vi "Main UI - Cylinder.vi"() -> ()   [LabVIEW 2015]
doc: "User interface for 64 pressure multiplexer system designed by Paul Nathan, 02/2016"
uses:
  Ctls/System status.ctl
  Ctls/Environmental state values.ctl
  Ctls/Inertial state values.ctl
  Ctls/AccelGyro constants.ctl
  Ctls/Pressure sensor constants.ctl
  Ctls/Cmd str.ctl
  Ctls/All state values (for datalog).ctl
  Ctls/Data values, Mode 0 (for datalog).ctl
  Ctls/Data values, Mode 1 (for datalog).ctl
panel:
  in  "Main tabs":T1(tab)
  out "ASCII done":bool caption="Done"
  in  "Write ASCII datalog":bool
  in  "Datalog name (without extension)":string="Log001"
  in  "Write interval (s)":u32=10
  in  "Save data":bool
  in  "Datalog directory":path=path "C:/Datalogs"
  out "ACK 8":bool caption="ACK"
  out "ACK 7":bool caption="ACK"
  out "ACK 6":bool caption="ACK"
  out "AccelGyro constants":T2={"gyrRange"=125.0, "accRange"=2.0, "gx offset"=0.0, "gy offset"=0.0, "gz offset"=0.0, "ax offset"=0.0, "ay offset"=0.0, "az offset"=0.0, "axyz scale"=1.0} {"axyz scale" format="%#_4f"; "az offset" format="%#_4f"; "ay offset" format="%#_4f"; "ax offset" format="%#_4f"; "gz offset" format="%#_4f"; "gy offset" format="%#_4f"; "gx offset" format="%#_4f"; "gyrRange" format="%#_4f"; "accRange" format="%#_4f"}
  out "Faulty sensors":i32[](array[numeric])
  out "ACK 5":bool caption="ACK"
  in  "Stop UI":bool
  out "Active sensors":i32[](array[numeric])
  in  "Refresh sys. status":bool
  out "ACK 4":bool caption="ACK"
  in  "Apply settings 3":bool caption="Apply settings"
  in  "Gyro. rate (Hz)":u8(ring) items=["6.25", "12.5", "25", "50", "100", "200", "400", "800", "1600", "3200"]
  in  "Gyro. range (dps)":u8(ring) items=["+/- 125", "+/- 250", "+/- 500", "+/- 1000", "+/- 2000"]
  in  "Accel. rate (Hz)":u8(ring)=1 items=["3.125", "6.25", "12.5", "25", "50", "100", "200", "400", "800", "1600"]
  in  "Accel. range (g)":u8(ring) items=["+/- 2", "+/- 4", "+/- 8", "+/- 16"]
  out "Inertial state values":T3 {"w_z (dps)" format="%#_4f"; "a_y (g)" format="%#_4f"; "a_z (g)" format="%#_4f"; "w_y (dps)" format="%#_4f"; "a_x (g)" format="%#_4f"; "Sensor temp. (degC)" format="%#.2f"; "w_x (dps)" format="%#_4f"}
  out "Environmental state values":T4 {"Dew point (degC)" format="%#.2f"; "Density (kg/m^3)" format="%#.3f"; "Pressure alt. (m)" format="%#.2f"; "Density alt. (m)" format="%#.2f"; "Rel. Humidity (%)" format="%#.2f"; "P_atmos (Pa)" format="%#_6f"; "Sensor temp. (degC)" format="%#.2f"; "Thermistor (degC)" format="%#.2f"}
  out "System status":T5
  out "ACK 3":bool caption="ACK"
  in  "Apply settings 2":bool caption="Apply setting"
  in  "Max. num. sensors (override)":u8=64 max=64
  out "ACK 1":bool caption="ACK"
  in  "Env. period (ms)":i32=1000 min=0
  in  "Data mode":u8(ring) items=["P", "P & T"]
  out "ACK 2":bool caption="ACK"
  in  "Apply settings 1":bool caption="Apply settings"
  in  "Data rate (Hz)":dbl=100.0
  in  "Reset":bool
  in  "Main Power":bool
  in  "Serial port":refnum<visa-resource-name>="COM1"
  out "Error":errorcluster
  out "L_data (bytes)":u16
  out "Serial no.":u16 format="%04x"
  out "Active pressure sensor constants":T6[](array[typedef])
  in  "d.p":i16=4
  in  "Wait for HW trigger":bool
  out "Clock drift":bool
  in  "Display rate (Hz)":dbl=100.0 min=0.0
  in  "N samples":u32=1000
  in  "Finite samples":bool
  out "Sensor temperatures time trace (Mode \"P & T\" only)":sgl[][](graph)
  out "Pressures time trace":sgl[][](graph)
  in  "Stop streaming":bool
  in  "Start streaming":bool
  out "Stale samples flag":u8[][](graph)
  out "Samples acquired":u32
  out "ok":bool
  out "Fx (N)":sgl format="%#_4g"
  out "Fy (N)":sgl format="%#_4g"
  in  "Filename (full path)":path=path "C:/Datalogs/Cp_snapshot_001.txt"
  in  "Snapshot":bool
  out "Cp distribution (time averaged)":cluster{"x/c flap (sorted)":sgl[], sgl[]}[](graph)
  out "Uref (m/s)":sgl format="%#_4g"
  # "[time averaged at display rate]"
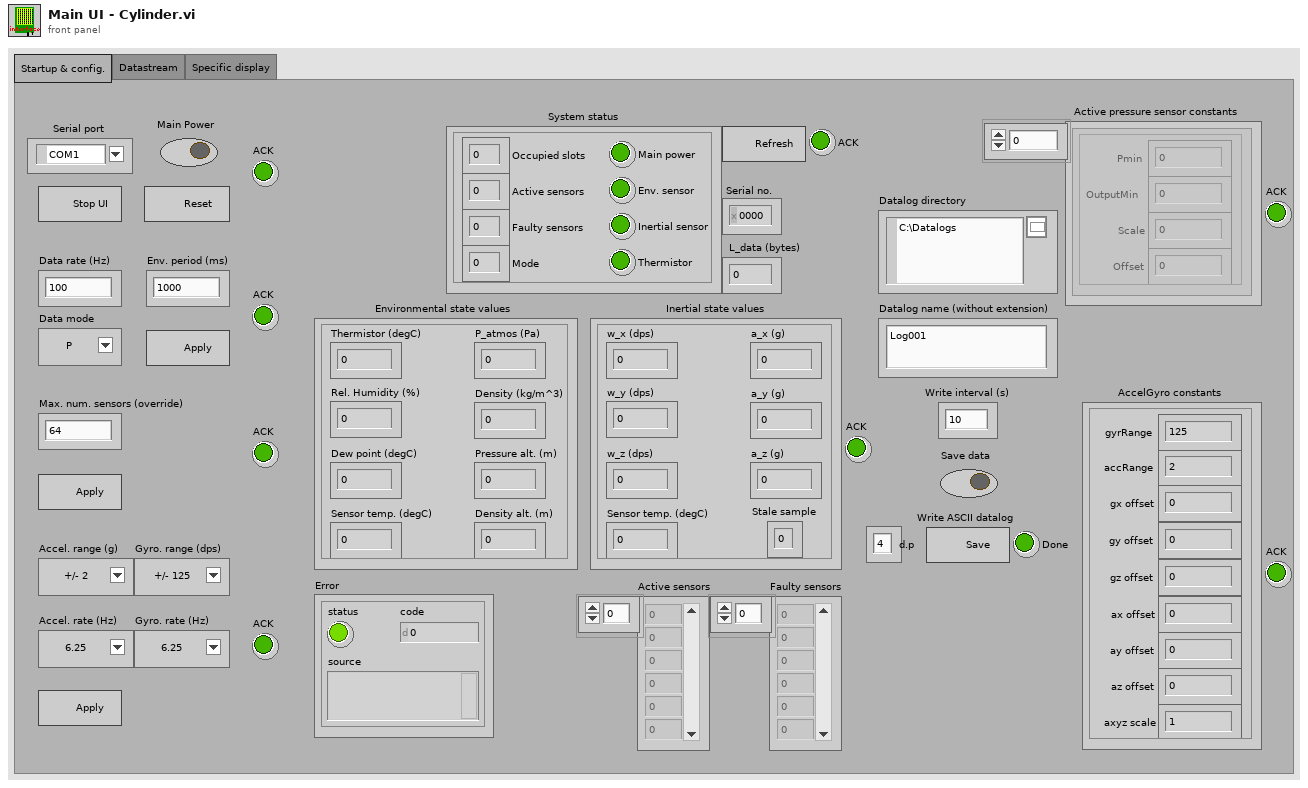
[diagram p1: front panel]
types:
  T1 = enum32{"Startup & config.", "Datastream", "Specific display"}
  T2 = typedef "AccelGyro constants.ctl" = cluster{"gyrRange":sgl, "accRange":sgl, "gx offset":sgl, "gy offset":sgl, "gz offset":sgl, "ax offset":sgl, "ay offset":sgl, "az offset":sgl, "axyz scale":sgl}
  T3 = typedef "Inertial state values.ctl" = cluster{"w_x (dps)":sgl, "w_y (dps)":sgl, "w_z (dps)":sgl, "a_x (g)":sgl, "a_y (g)":sgl, "a_z (g)":sgl, "Stale sample":u8, "Sensor temp. (degC)":sgl}
  T4 = typedef "Environmental state values.ctl" = cluster{"Thermistor (degC)":sgl, "Sensor temp. (degC)":sgl, "P_atmos (Pa)":sgl, "Rel. Humidity (%)":sgl, "Density (kg/m^3)":sgl, "Dew point (degC)":sgl, "Pressure alt. (m)":sgl, "Density alt. (m)":sgl}
  T5 = typedef "System status.ctl" = cluster{"Main power":bool, "Occupied slots":u8, "Active sensors":u8, "Faulty sensors":u8, "Env. sensor":bool, "Inertial sensor":bool, "Thermistor":bool, "Mode":u8}
  T6 = typedef "Pressure sensor constants.ctl" = cluster{"Pmin":sgl, "OutputMin":sgl, "Scale":sgl, "Offset":sgl}
  T7 = typedef "Cmd str.ctl" = string
  T8 = typedef "All state values (for datalog).ctl" = cluster{"Time Stamp":timestamp, "dt (ms)":i32, "Environmental state values":T4, "Inertial state values":T3}
  T9 = typedef "Data values, Mode 1 (for datalog).ctl" = cluster{"Time Stamp":timestamp, "dt (us)":sgl, "dt_warn":u8, "Pressures":sgl[], "Die temps.":sgl[], "Statuses":u8[]}
  T10 = typedef "Data values, Mode 0 (for datalog).ctl" = cluster{"Time Stamp":timestamp, "dt (us)":sgl, "dt_warn":u8, "Pressures":sgl[], "Statuses":u8[]}
  T11 = enum8{"Enabled", "Disabled", "Disabled and Grayed Out"}
  T12 = typedef "EEPROM page.ctl" = cluster{"Pmin (Pa)":sgl, "Pmax (Pa)":sgl, "maxCount":u16, "minCount":u16, "Poffset (Pa)":sgl}
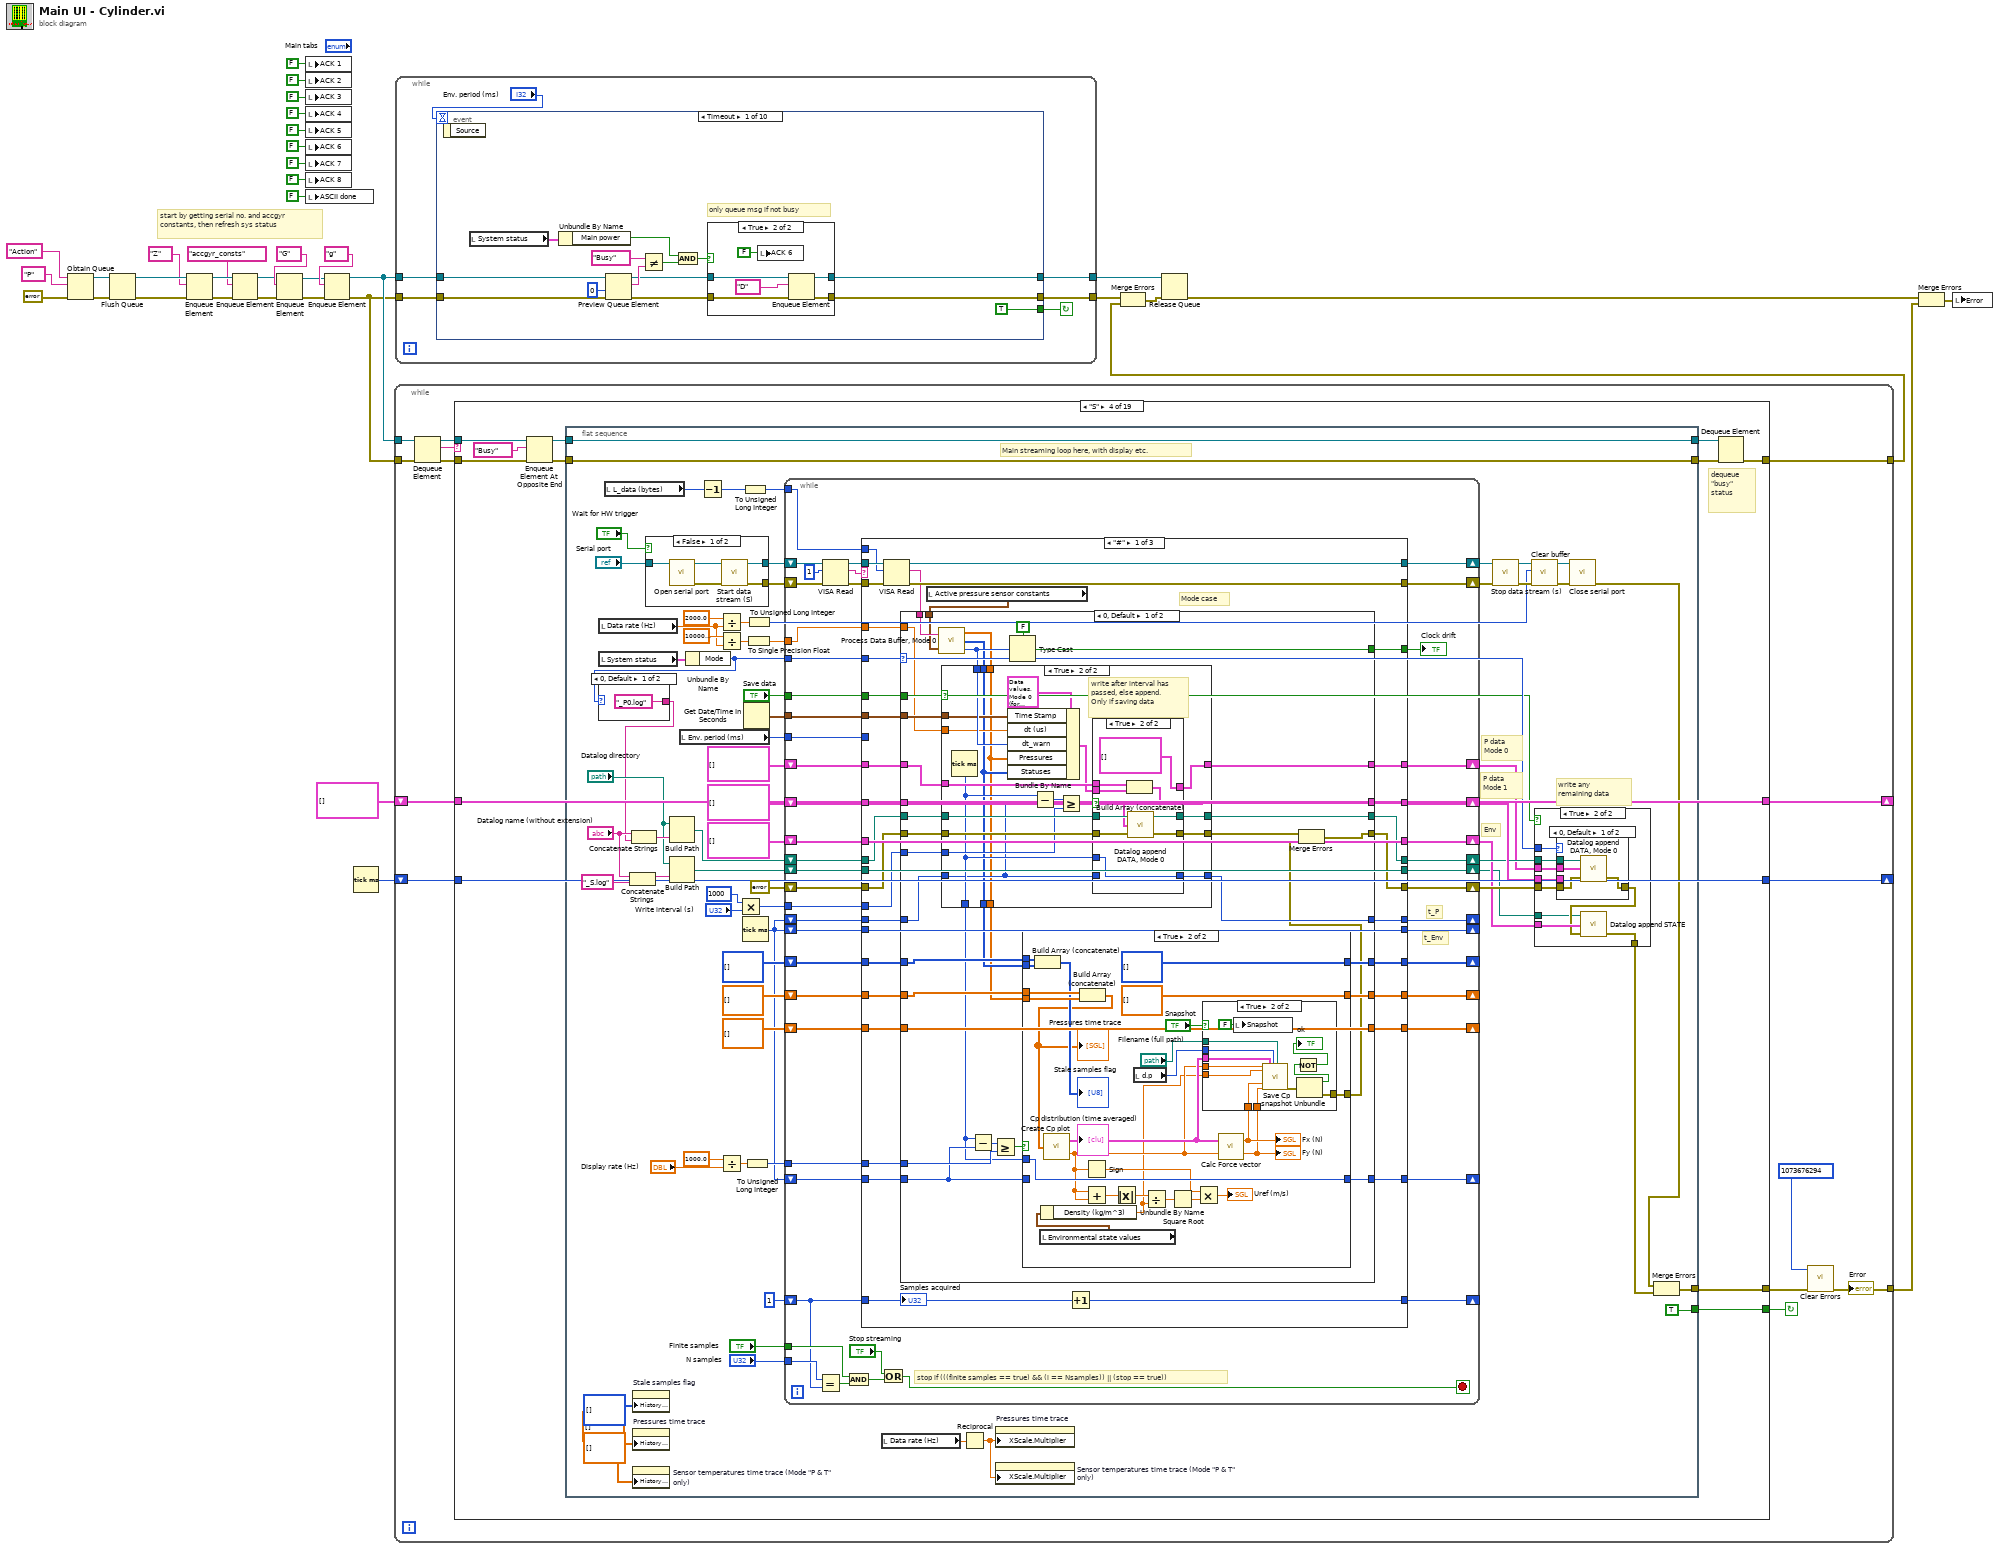
[diagram p0: block diagram]
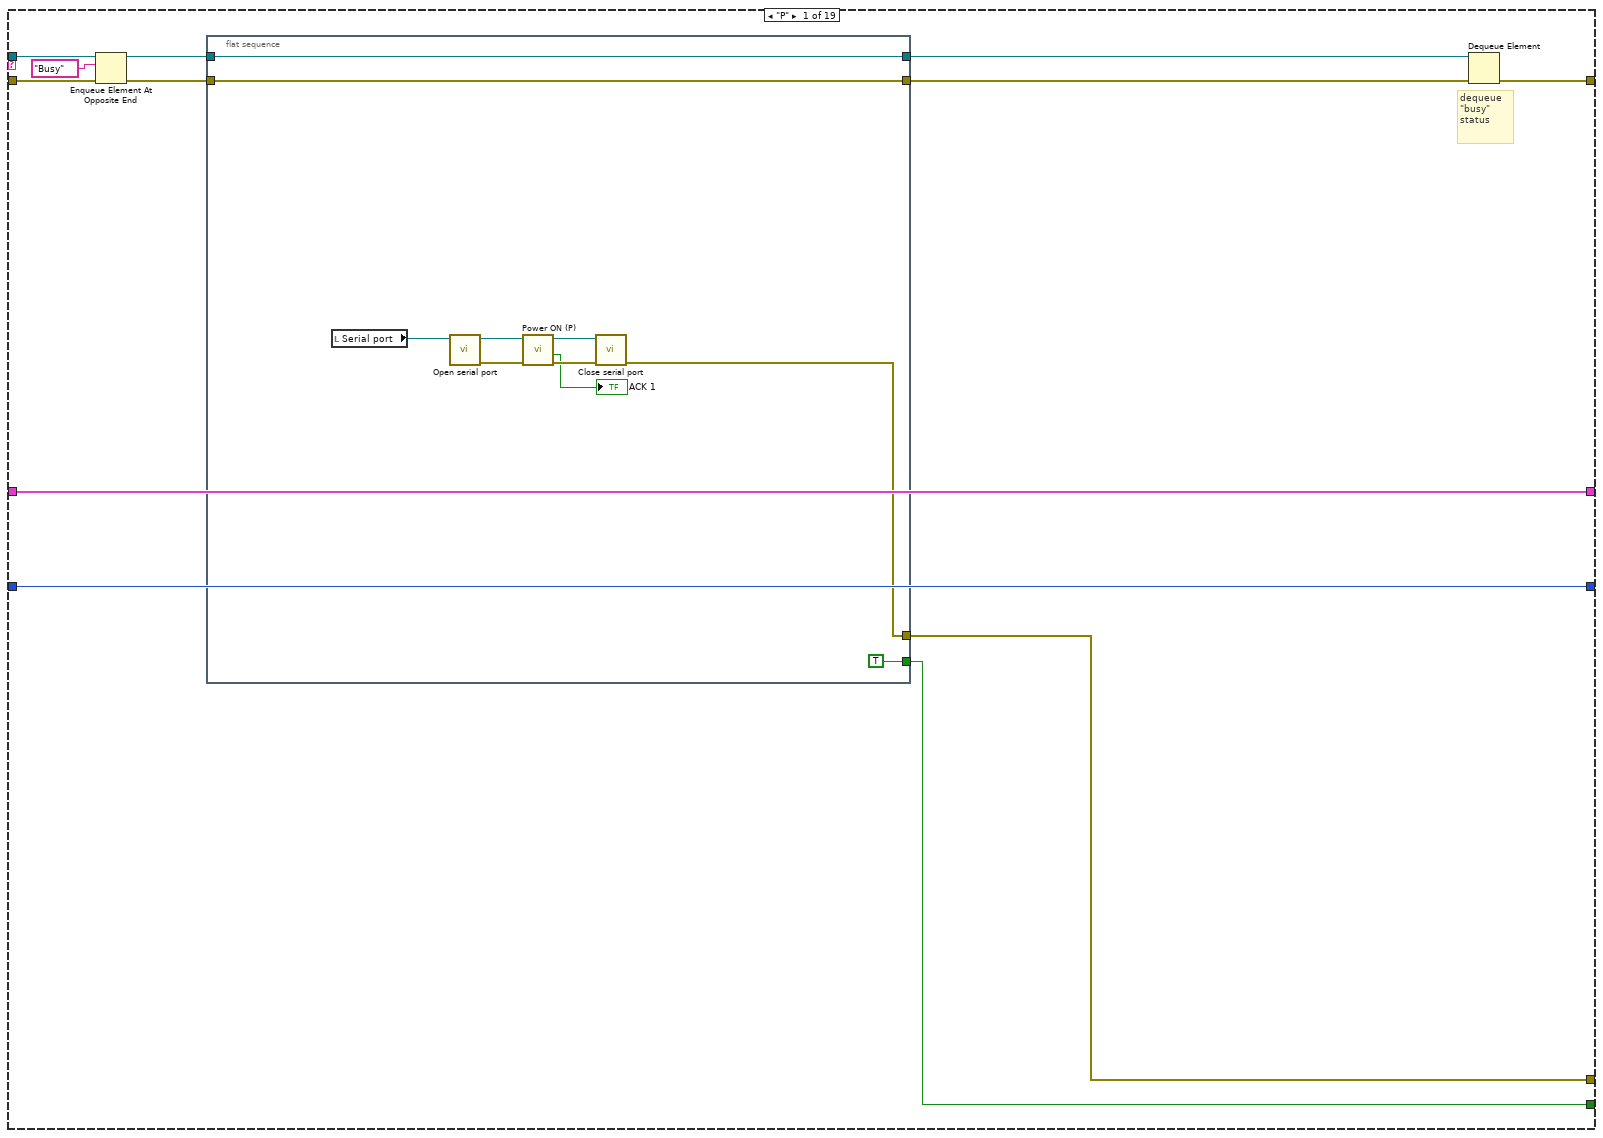
[diagram p2: hidden frame]
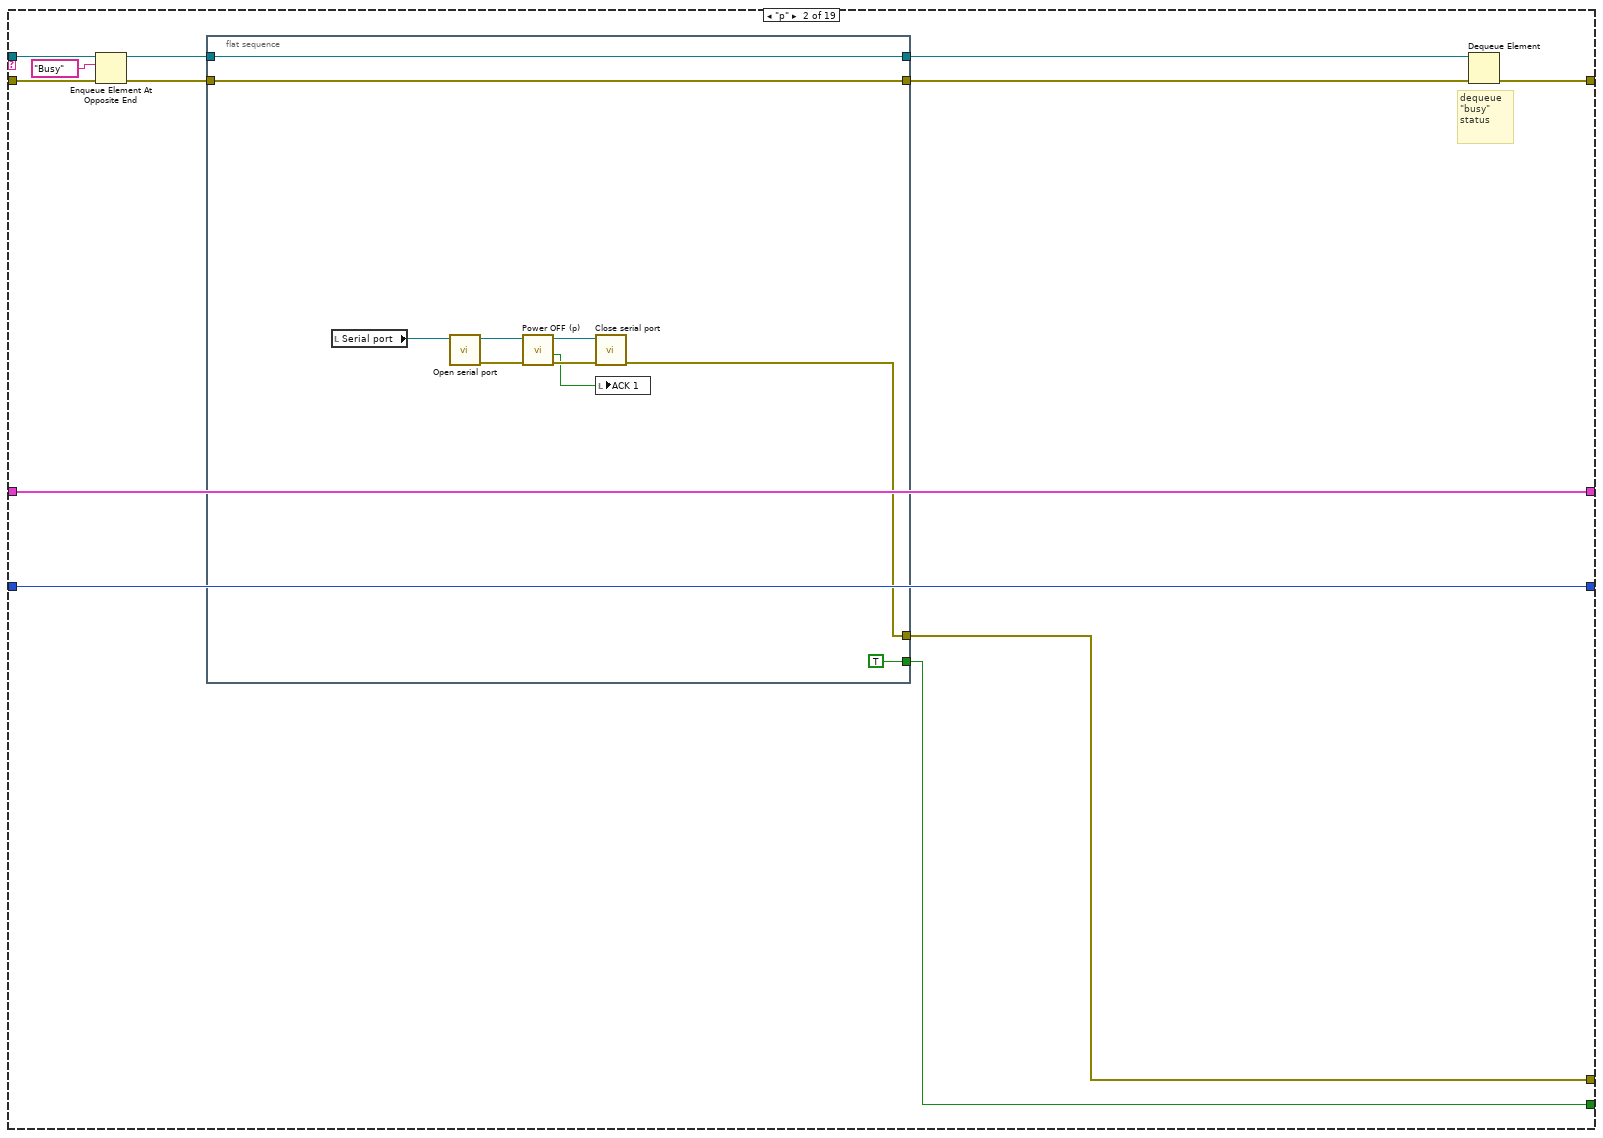
[diagram p3: hidden frame]
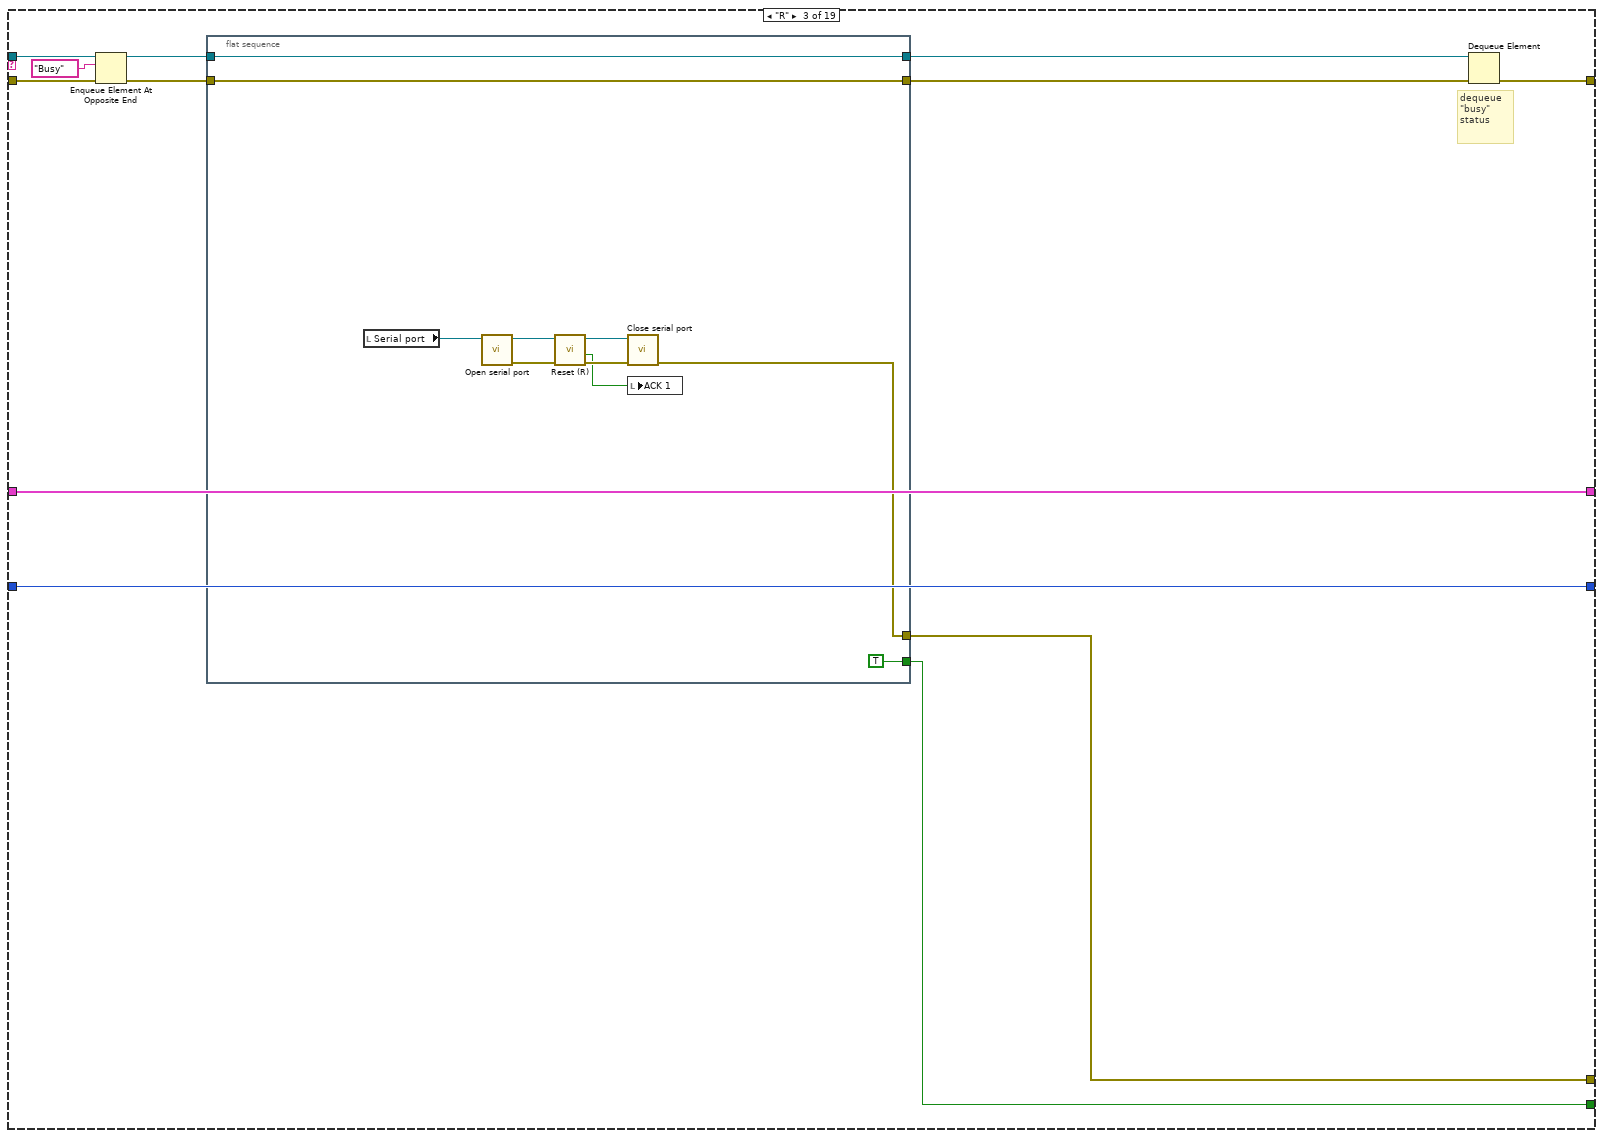
[diagram p4: hidden frame]
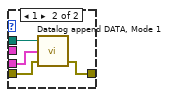
[diagram p6: hidden frame]
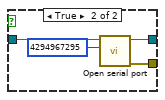
[diagram p7: hidden frame]
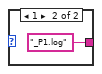
[diagram p8: hidden frame]
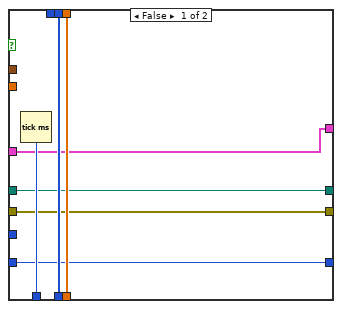
[diagram p9: hidden frame]
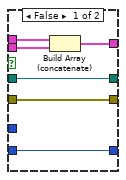
[diagram p10: hidden frame]
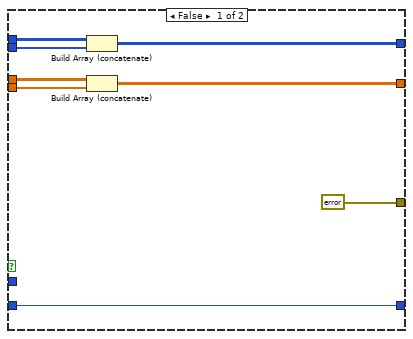
[diagram p11: hidden frame]
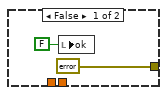
[diagram p12: hidden frame]
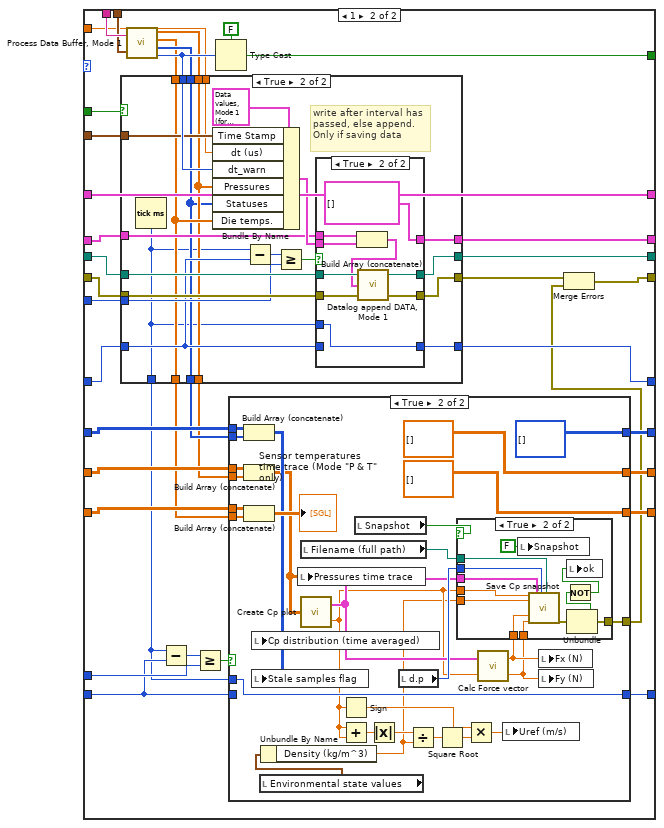
[diagram p13: hidden frame]
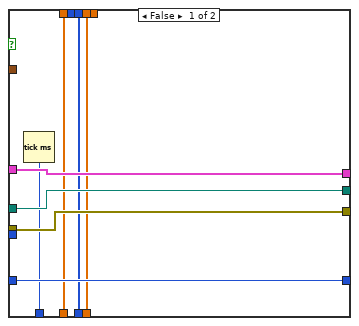
[diagram p14: hidden frame]
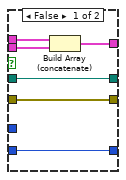
[diagram p15: hidden frame]
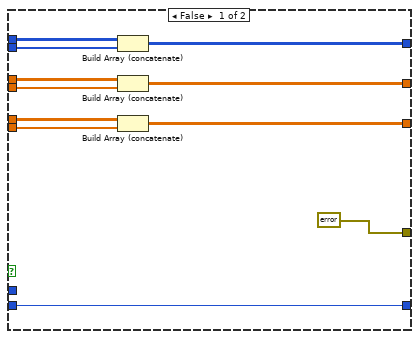
[diagram p16: hidden frame]
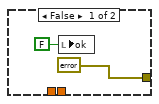
[diagram p17: hidden frame]
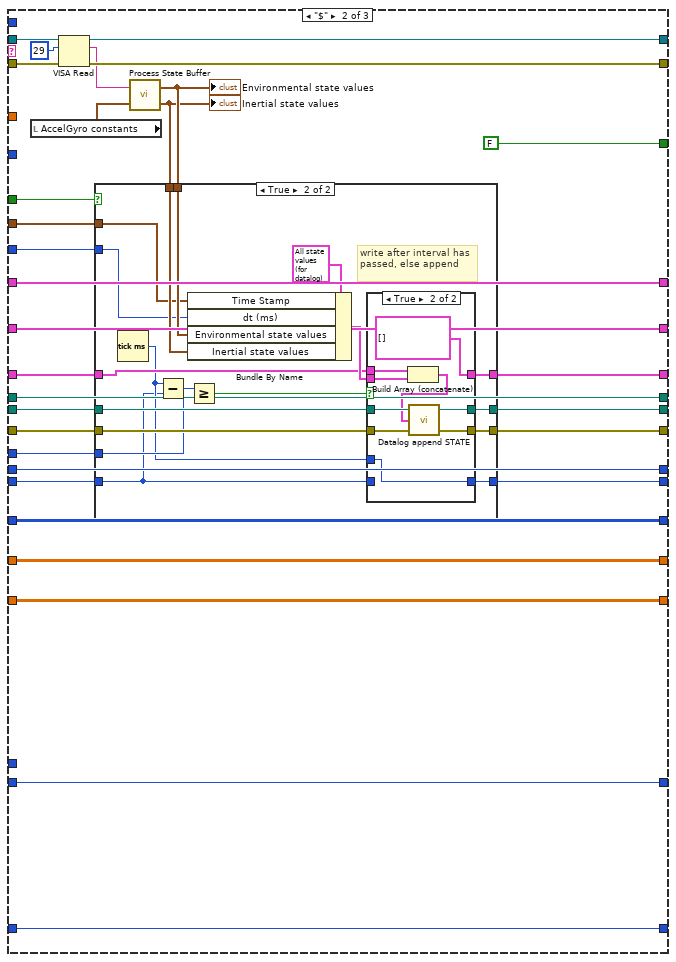
[diagram p18: hidden frame]
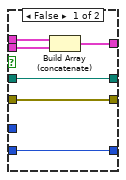
[diagram p20: hidden frame]
diagram:
  # "start by getting serial no. and accgyr constants, then refresh sys status"
  n1 = Obtain Queue(name (unnamed)="Action", element data type=T7 "P" ("Cmd"), error in (no error)=errorcluster {"status"=FALSE, "code"=0, "source"=""}) -> (queue out=w36:refnum<queue>, error out=w35:errorcluster)  [unwired: 2 in, 1 out]
  n2 = Flush Queue(queue=w36, error in (no error)=w35) -> (queue out=w28:refnum<queue>, error out=w27:errorcluster)  [unwired: 1 out]
  n3 = Enqueue Element(queue=w28, element=T7 "Z", error in (no error)=w27) -> (queue out=w25:refnum<queue>, error out=w24:errorcluster)  [unwired: 1 in, 1 out]
  n4 = Enqueue Element(queue=w25, element=T7 "accgyr_consts", error in (no error)=w24) -> (queue out=w12:refnum<queue>, error out=w11:errorcluster)  [unwired: 1 in, 1 out]
  n5 = Enqueue Element(queue=w12, element=T7 "G" ("Cmd"), error in (no error)=w11) -> (queue out=w14:refnum<queue>, error out=w15:errorcluster)  [unwired: 1 in, 1 out]
  n6 = local write "ACK 1"(FALSE ("ACK 8")) -> ()
  n7 = local write "ACK 2"(FALSE ("ACK 6")) -> ()
  n8 = local write "ACK 3"(FALSE ("ACK 8")) -> ()
  n9 = local write "ACK 4"(FALSE ("Done")) -> ()
  n10 = local write "ACK 5"(FALSE ("ACK 8")) -> ()
  n11 = local write "ACK 6"(FALSE ("ACK 6")) -> ()
  n12 = local write "ACK 7"(FALSE ("ACK 6")) -> ()
  n13 = local write "ACK 8"(FALSE ("ACK 8")) -> ()
  n14 = local write "ASCII done"(FALSE ("Done")) -> ()
  n15 = Enqueue Element(queue=w14, element=T7 "g" ("Cmd"), error in (no error)=w15) -> (queue out=w10:refnum<queue>, error out=w9:errorcluster)  [unwired: 1 in, 1 out]
  n16 = Tick Count (ms)() -> (millisecond timer value=w20:u32)
  n17 = while {
    tunnel: w9 -> [w50]
    tunnel: w10 -> [w51]
    tunnel: [w47] -> w30
    shift-right: [w44] -> _
    shift-left: T8[] [] -> [w43]
    tunnel: [w38] -> w18
    shift-right: [w41] -> _
    shift-left: w20 -> [w42]
    stop <- w46 continue-if-true
    n18 = Dequeue Element(queue=w51, error in (no error)=w50) -> (queue out=w49:refnum<queue>, element=w45:T7, error out=w48:errorcluster)  [unwired: 1 in, 1 out]
    n19 = case shown="\"S\"" w45 {
      tunnel: w49 -> [w63 w85 w107 w129 w664 w689 w713 w737 w761 w789 w826 w848 w870 w909 w933 w1006 w1038 w1066 _]
      tunnel: w48 -> [w62 w84 w106 w128 w663 w688 w712 w736 w760 w788 w825 w847 w869 w908 w932 w1005 w1037 w1065 w1135]
      tunnel: [w57 w79 w101 w123 w658 w683 w707 w731 w755 w783 w820 w842 w864 w903 w927 w1000 w1032 w1060 w1135] -> w47
      tunnel: [w56 w78 w100 w122 w657 w682 w706 w730 w754 w782 w819 w841 w863 w902 w926 w999 w1031 w1059 FALSE] -> w46
      tunnel: [w55 w77 w99 w121 w656 w681 w705 w729 w753 w781 w818 w840 w862 w901 w925 w998 w1030 w1058 errorcluster {"status"=FALSE, "code"=0, "source"=""} ("Error out")] -> w39
      tunnel: [w53 w75 w97 w118 w654 w679 w703 w727 w751 w779 w816 w838 w860 w899 w923 w995 w1028 w1056 w1132] -> w44
      tunnel: w43 -> [w53 w75 w97 w118 w654 w679 w703 w727 w751 w779 w816 w838 w860 w899 w922 w995 w1028 w1056 w1132]
      tunnel: w42 -> [w52 w74 w96 w119 w653 w678 w702 w726 w750 w778 w815 w837 w859 w898 w921 w996 w1027 w1055 w1131]
      tunnel: [w52 w74 w96 w119 w653 w678 w702 w726 w750 w778 w815 w837 w859 w898 w920 w996 w1027 w1055 w1131] -> w41
      frame "P" {
        # "dequeue \"busy\" status"
        n20 = Enqueue Element At Opposite End(queue=w63, element=T7 "Busy" ("Cmd"), error in (no error)=w62) -> (queue out=w61:refnum<queue>, error out=w60:errorcluster)  [unwired: 1 in, 1 out]
        n21 = flat-sequence {
          tunnel: w61 -> [w73]
          tunnel: w60 -> [w72]
          tunnel: [w73] -> w59
          tunnel: [w72] -> w58
          tunnel: [TRUE] -> w56
          tunnel: [w66] -> w55
          frame #0 {
            n22 = local read "Serial port"() -> (w65:refnum<visa-resource-name>)
            n23 = call "Open serial port.vi"("VISA resource name"=w65) -> ("Error out"=w69:errorcluster, "VISA resource name out"=w70:refnum<visa-resource-name>)  [unwired: 9 in]
            n24 = call "Power ON (P).vi"("Error In"=w69, "VISA resource name in"=w70) -> ("Error out"=w68:errorcluster, "ACK"=→"ACK 1":bool, "VISA resource name out"=w67:refnum<visa-resource-name>)  [unwired: 7 in]
            n25 = call "Close serial port.vi"("Error in"=w68, "VISA resource name"=w67) -> ("Error out"=w66:errorcluster)  [unwired: 9 in]
          }
        }
        n26 = Dequeue Element(queue=w59, error in (no error)=w58) -> (error out=w57:errorcluster)  [unwired: 1 in, 3 out]
      }
      frame "p" {
        # "dequeue \"busy\" status"
        n27 = Enqueue Element At Opposite End(queue=w85, element=T7 "Busy" ("Cmd"), error in (no error)=w84) -> (queue out=w83:refnum<queue>, error out=w82:errorcluster)  [unwired: 1 in, 1 out]
        n28 = flat-sequence {
          tunnel: w83 -> [w95]
          tunnel: w82 -> [w94]
          tunnel: [w95] -> w81
          tunnel: [w94] -> w80
          tunnel: [TRUE] -> w78
          tunnel: [w88] -> w77
          frame #0 {
            n29 = local read "Serial port"() -> (w86:refnum<visa-resource-name>)
            n30 = call "Open serial port.vi"("VISA resource name"=w86) -> ("Error out"=w91:errorcluster, "VISA resource name out"=w92:refnum<visa-resource-name>)  [unwired: 9 in]
            n31 = call "Power OFF (p).vi"("Error In"=w91, "VISA resource name in"=w92) -> ("Error out"=w90:errorcluster, "ACK"=w87:bool, "VISA resource name out"=w89:refnum<visa-resource-name>)  [unwired: 7 in]
            n32 = call "Close serial port.vi"("Error in"=w90, "VISA resource name"=w89) -> ("Error out"=w88:errorcluster)  [unwired: 9 in]
            n33 = local write "ACK 1"(w87) -> ()
          }
        }
        n34 = Dequeue Element(queue=w81, error in (no error)=w80) -> (error out=w79:errorcluster)  [unwired: 1 in, 3 out]
      }
      frame "R" {
        # "dequeue \"busy\" status"
        n35 = Enqueue Element At Opposite End(queue=w107, element=T7 "Busy" ("Cmd"), error in (no error)=w106) -> (queue out=w105:refnum<queue>, error out=w104:errorcluster)  [unwired: 1 in, 1 out]
        n36 = flat-sequence {
          tunnel: w105 -> [w117]
          tunnel: w104 -> [w116]
          tunnel: [w117] -> w103
          tunnel: [w116] -> w102
          tunnel: [TRUE] -> w100
          tunnel: [w112] -> w99
          frame #0 {
            n37 = local read "Serial port"() -> (w110:refnum<visa-resource-name>)
            n38 = call "Open serial port.vi"("VISA resource name"=w110) -> ("Error out"=w108:errorcluster, "VISA resource name out"=w109:refnum<visa-resource-name>)  [unwired: 9 in]
            n39 = call "Reset (R).vi"("Error In"=w108, "VISA resource name in"=w109) -> ("Error out"=w114:errorcluster, "ACK"=w111:bool, "VISA resource name out"=w113:refnum<visa-resource-name>)  [unwired: 7 in]
            n40 = call "Close serial port.vi"("Error in"=w114, "VISA resource name"=w113) -> ("Error out"=w112:errorcluster)  [unwired: 9 in]
            n41 = local write "ACK 1"(w111) -> ()
          }
        }
        n42 = Dequeue Element(queue=w103, error in (no error)=w102) -> (error out=w101:errorcluster)  [unwired: 1 in, 3 out]
      }
      frame "S" {
        # "dequeue \"busy\" status"
        n43 = Enqueue Element At Opposite End(queue=w129, element=T7 "Busy" ("Cmd"), error in (no error)=w128) -> (queue out=w127:refnum<queue>, error out=w126:errorcluster)  [unwired: 1 in, 1 out]
        n44 = flat-sequence {
          tunnel: w127 -> [w197]
          tunnel: w126 -> [w196]
          tunnel: [w197] -> w125
          tunnel: [w196] -> w124
          tunnel: [TRUE] -> w122
          tunnel: [w183] -> w121
          frame #0 {
            # "Env"
            # "P data Mode 1"
            # "P data Mode 0"
            # "write any remaining data"
            # "Main streaming loop here, with display etc."
            n45 = local read "Data rate (Hz)"() -> (w158:dbl)
            n46 = local read "System status"() -> (w155:T5)
            n47 = local read "L_data (bytes)"() -> (w162:u16)
            n48 = Concatenate Strings("Datalog name (without extension)", "_S.log" ("string")) -> (w169:string)
            n49 = property on="Stale samples flag" class="WFChart (strict)"("History Data"=u8[][] []) -> ()  [unwired: 2 in, 2 out]
            n50 = property on="Pressures time trace" class="WFChart (strict)"("History Data"=sgl[][] []) -> ()  [unwired: 2 in, 2 out]
            n51 = property on="Sensor temperatures time trace (Mode \"P & T\" only)" class="WFChart (strict)"("History Data"=sgl[][] []) -> ()  [unwired: 2 in, 2 out]
            n52 = case shown="False" "Wait for HW trigger" {
              tunnel: [w218 w222] -> w194
              tunnel: [w217 w223] -> w193
              tunnel: "Serial port" -> [w216 w224]
              frame False {
                n53 = call "Open serial port.vi"("VISA resource name"=w216) -> ("Error out"=w219:errorcluster, "VISA resource name out"=w220:refnum<visa-resource-name>)  [unwired: 9 in]
                n54 = call "Start data stream (S).vi"("VISA resource name in"=w220, "Error In"=w219) -> ("VISA resource name out"=w217:refnum<visa-resource-name>, "Error out"=w218:errorcluster)  [unwired: 7 in]
              }
              frame True {
                n55 = call "Open serial port.vi"("timeout (ms)"=u32 4294967295, "VISA resource name"=w224) -> ("Error out"=w222:errorcluster, "VISA resource name out"=w223:refnum<visa-resource-name>)  [unwired: 8 in]
              }
            }
            n56 = Build Path(base path="Datalog directory", name or relative path=w169) -> (appended path=w165:path)
            n57 = local read "Env. period (ms)"() -> (w160:i32)
            n58 = Unbundle By Name(w155) -> ("Mode"=w140:u8)
            n59 = case shown="0, Default" w140 {
              tunnel: ["_P0.log" ("string") "_P1.log" ("string")] -> w154
              frame 0, Default {
              }
              frame 1 {
              }
            }
            n60 = Concatenate Strings("Datalog name (without extension)", w154) -> (w177:string)
            n61 = Build Path(base path="Datalog directory", name or relative path=w177) -> (appended path=w166:path)
            n62 = Decrement(x=w162) -> (x-1=w144:u16)
            n63 = Divide(x=2000.0 ("y"), y=w158) -> (x/y=w186:dbl)
            n64 = Divide(x=1000000.0 ("y"), y=w158) -> (x/y=w157:dbl)
            n65 = Divide(x=1000.0, y="Display rate (Hz)") -> (x/y=w175:dbl)
            n66 = Multiply(x=u32 1000, y="Write interval (s)") -> (x*y=w179:u32)
            n67 = To Unsigned Long Integer(number=w144) -> (unsigned 32bit integer=w161:u32)
            n68 = Tick Count (ms)() -> (millisecond timer value=w145:u32)
            n69 = Get Date/Time In Seconds() -> (seconds since 1Jan1904=w192:timestamp)
            n70 = To Unsigned Long Integer(number=w175) -> (unsigned 32bit integer=w172:u32)
            n71 = To Unsigned Long Integer(number=w186) -> (unsigned 32bit integer=w185:u32)
            n72 = To Single Precision Float(number=w157) -> (single precision float=w156:sgl)
            n73 = while {
              shift-right: [w269] -> w189
              shift-left: w193 -> [w274]
              shift-right: [w268] -> w190
              shift-left: w194 -> [w275]
              tunnel: w192 -> [w267]
              shift-right: [w266] -> w142
              shift-left: errorcluster {"status"=FALSE, "code"=0, "source"=""} ("Error out") -> [w265]
              tunnel: "Finite samples" -> [w262]
              tunnel: "N samples" -> [w264]
              tunnel: "Save data" -> [w258]
              shift-right: [w256] -> w136
              shift-left: w165 -> [w257]
              shift-right: [w255] -> w138
              shift-left: T8[] [] -> [w254]
              tunnel: w179 -> [w252]
              shift-right: [w247] -> _
              shift-left: w145 -> [w253]
              tunnel: w172 -> [w236]
              shift-right: [w250] -> w141
              shift-left: w166 -> [w251]
              shift-right: [w248] -> _
              shift-left: w145 -> [w249]
              shift-right: [w243] -> w143
              shift-left: T9[] [] -> [w245]
              shift-right: [w244] -> w139
              shift-left: T10[] [] -> [w246]
              tunnel: w161 -> [w242]
              tunnel: w160 -> [w241]
              tunnel: w156 -> [w240]
              tunnel: w140 -> [w229]
              shift-right: [w238] -> _
              shift-left: w145 -> [w237]
              shift-right: [w235] -> _
              shift-left: sgl[][] [] -> [w232]
              shift-right: [w234] -> _
              shift-left: u8[][] [] -> [w233]
              shift-right: [w231] -> _
              shift-left: sgl[][] [] -> [w230]
              shift-right: [w228] -> _
              shift-left: u32 1 ("x") -> [w227]
              stop <- w259 stop-if-true
              # "t_Env"
              # "t_P"
              # "stop if (((finite samples == true) && (i == Nsamples)) || (stop == true))"
              n74 = Equal?(x=w264, y=w227) -> (x = y?=w263:bool)
              n75 = VISA Read(VISA resource name=w274, byte count=u32 1, error in (no error)=w275) -> (VISA resource name out=w271:refnum<visa-resource-name>, read buffer=w272:string, error out=w270:errorcluster)  [unwired: 1 out]
              n76 = And(x=w262, y=w263) -> (x .and. y?=w260:bool)
              n77 = case shown="\"#\"" w272 {
                tunnel: w271 -> [w310 w598 w652]
                tunnel: w270 -> [w309 w597 w651]
                tunnel: [w307 w595 w652] -> w269
                tunnel: [w306 w596 w651] -> w268
                tunnel: w267 -> [w303 w592 _]
                tunnel: [w289 w591 w650] -> w266
                tunnel: w265 -> [w299 w590 w650]
                tunnel: w258 -> [w278 w589 _]
                tunnel: w257 -> [w312 w588 w649]
                tunnel: [w312 w587 w649] -> w256
                tunnel: [w311 w586 w648] -> w255
                tunnel: w254 -> [w311 w585 w648]
                tunnel: w253 -> [w294 w578 w645]
                tunnel: w252 -> [w296 w584 _]
                tunnel: [w295 w583 w646] -> w248
                tunnel: w251 -> [w300 w580 w647]
                tunnel: [w288 w580 w647] -> w250
                tunnel: w249 -> [w295 w579 w646]
                tunnel: [w298 w578 w645] -> w247
                tunnel: w246 -> [w302 w577 w643]
                tunnel: w245 -> [w291 w576 w644]
                tunnel: [w301 w577 w643] -> w244
                tunnel: [w290 w576 w644] -> w243
                tunnel: w242 -> [w308 _ _]
                tunnel: w241 -> [_ w575 _]
                tunnel: w240 -> [w297 _ _]
                tunnel: [w293 FALSE ("Clock drift") FALSE ("Clock drift")] -> w239
                tunnel: w229 -> [w292 _ _]
                tunnel: [w287 w573 w641] -> w238
                tunnel: w237 -> [w286 w573 w641]
                tunnel: w236 -> [w285 _ _]
                tunnel: [w284 w571 w639] -> w235
                tunnel: w232 -> [w283 w571 w639]
                tunnel: [w282 w572 w640] -> w234
                tunnel: w233 -> [w281 w572 w640]
                tunnel: [w280 w570 w638] -> w231
                tunnel: w230 -> [w279 w570 w638]
                tunnel: [w277 w569 w637] -> w228
                tunnel: w227 -> [w276 w569 w637]
                frame "#" {
                  # "Mode case"
                  n78 = VISA Read(VISA resource name=w310, byte count=w308, error in (no error)=w309) -> (VISA resource name out=w307:refnum<visa-resource-name>, read buffer=w305:string, error out=w306:errorcluster)  [unwired: 1 out]
                  n79 = local read "Active pressure sensor constants"() -> (w304:T6[])
                  n80 = case shown="0, Default" w292 {
                    tunnel: w305 -> [w346 w471]
                    tunnel: w304 -> [w345 w470]
                    tunnel: w303 -> [w342 w467]
                    tunnel: w302 -> [w341 w472]
                    tunnel: [w340 w472] -> w301
                    tunnel: w300 -> [w339 w466]
                    tunnel: w299 -> [w338 w465]
                    tunnel: [w337 w464] -> w298
                    tunnel: w297 -> [w336 w463]
                    tunnel: w296 -> [w335 w462]
                    tunnel: w294 -> [w320 w461]
                    tunnel: [w334 w460] -> w293
                    tunnel: w291 -> [w347 w459]
                    tunnel: [w347 w458] -> w290
                    tunnel: [w313 w437] -> w289
                    tunnel: [w333 w457] -> w288
                    tunnel: [w332 w451] -> w287
                    tunnel: w286 -> [w329 w447]
                    tunnel: w285 -> [w331 w448]
                    tunnel: [w326 w455] -> w284
                    tunnel: w283 -> [w325 w453]
                    tunnel: [w323 w456] -> w282
                    tunnel: w281 -> [w322 w454]
                    tunnel: [w321 w445] -> w280
                    tunnel: w279 -> [w321 w443]
                    tunnel: w278 -> [w317 w442]
                    frame 0, Default {
                      n81 = call "Process Data Buffer, Mode 0.vi"("DATA_Buffer excluding '#' [1...N]"=w346, "P constants"=w345) -> ("Pressures"=w327:sgl[], "Statuses"=w324:u8[], "dt_warn"=w343:u8)
                      n82 = case shown="True" w317 {
                        tunnel: w343 -> [_ w372]
                        tunnel: w342 -> [_ w371]
                        tunnel: w341 -> [w349 w370]
                        tunnel: [w349 w368] -> w340
                        tunnel: w339 -> [w350 w367]
                        tunnel: w338 -> [w351 w366]
                        tunnel: [w348 w365] -> w337
                        tunnel: w336 -> [_ w364]
                        tunnel: w335 -> [_ w361]
                        tunnel: [w351 w360] -> w315
                        tunnel: [w350 w359] -> w333
                        tunnel: [w354 w358] -> w316
                        tunnel: w327 -> [w352 w355]
                        tunnel: w324 -> [w353 w356]
                        tunnel: w320 -> [w348 w357]
                        tunnel: [w353 w356] -> w319
                        tunnel: [w352 w355] -> w318
                        frame False {
                          n83 = Tick Count (ms)() -> (millisecond timer value=w354:u32)
                        }
                        frame True {
                          # "write after interval has passed, else append. Only if saving data"
                          n84 = Tick Count (ms)() -> (millisecond timer value=w358:u32)
                          n85 = Bundle By Name(cluster=T10 {"Time Stamp"=timestamp(3537581686.1176577 s since 1904-01-01), "dt (us)"=0.0, "dt_warn"=0, "Pressures"=[], "Statuses"=[]} ("P data (Mode 0)"), "Time Stamp"=w371, "dt (us)"=w364, "dt_warn"=w372, "Pressures"=w355, "Statuses"=w356) -> (w369:T10)
                          n86 = Subtract(x=w358, y=w357) -> (x-y=w363:u32)
                          n87 = Greater Or Equal?(x=w363, y=w361) -> (x >= y?=w362:bool)
                          n88 = case shown="True" w362 {
                            tunnel: [w375 w388] -> w360
                            tunnel: w366 -> [w375 w387]
                            tunnel: w367 -> [w376 w386]
                            tunnel: [w376 w385] -> w359
                            tunnel: w369 -> [w378 w384]
                            tunnel: w370 -> [w379 w383]
                            tunnel: [w377 T10[] []] -> w368
                            tunnel: w358 -> [_ w382]
                            tunnel: [w374 w382] -> w365
                            tunnel: w357 -> [w374 _]
                            frame False {
                              n89 = Build Array (concatenate)(w379, w378) -> (w377:T10[])
                            }
                            frame True {
                              n90 = Build Array (concatenate)(w383, w384) -> (w380:T10[])
                              n91 = call "Datalog append DATA, Mode 0.vi"("Datalog (Data) path"=w386, "Data (Mode 0)"=w380, "Error in"=w387) -> ("Path out"=w385:path, "Error out"=w388:errorcluster)  [unwired: 5 in]
                            }
                          }
                        }
                      }
                      n92 = Subtract(x=w316, y=w329) -> (x-y=w330:u32)
                      n93 = Greater Or Equal?(x=w330, y=w331) -> (x >= y?=w328:bool)
                      n94 = Type Cast(type=FALSE ("Clock drift"), x=w343) -> (*(type *) &x=w334:bool)
                      n95 = case shown="True" w328 {
                        tunnel: [w396 w421] -> w332
                        tunnel: w329 -> [w396 _]
                        tunnel: w316 -> [_ w421]
                        tunnel: w318 -> [w395 w419]
                        tunnel: [w394 sgl[][] []] -> w326
                        tunnel: w325 -> [w393 w420]
                        tunnel: w319 -> [w392 w416]
                        tunnel: [w391 u8[][] []] -> w323
                        tunnel: w322 -> [w390 w417]
                        tunnel: [errorcluster {"status"=FALSE, "code"=0, "source"=""} ("error out") w410] -> w314
                        frame False {
                          n96 = Build Array (concatenate)(w390, w392) -> (w391:u8[][])
                          n97 = Build Array (concatenate)(w393, w395) -> (w394:sgl[][])
                        }
                        frame True {
                          n98 = Build Array (concatenate)(w417, w416) -> (→"Stale samples flag":u8[][])
                          n99 = local read "Environmental state values"() -> (w408:T4)
                          n100 = Unbundle By Name(w408) -> ("Density (kg/m^3)"=w399:sgl)
                          n101 = Build Array (concatenate)(w420, w419) -> (w413:sgl[][])
                          "Pressures time trace" <- w413
                          n102 = call "Create Cp plot.vi"("Pressures in (cols = sensor, rows = time)"=w413) -> ("Cp against x/c"=w401:cluster{"x/c flap (sorted)":sgl[], sgl[]}[], "Pdyn ref (Pa)"=w400:sgl)
                          "Cp distribution (time averaged)" <- w401
                          n103 = Sign(1:w400) -> (0:w402:sgl)
                          n104 = Add(x=w400, y=w400) -> (x+y=w407:sgl)
                          n105 = Absolute Value(x=w407) -> (abs(x)=w405:sgl)
                          n106 = local read "d.p"() -> (w411:i16)
                          n107 = Divide(x=w405, y=w399) -> (x/y=w406:sgl)
                          n108 = Square Root(x=w406) -> (sqrt(x)=w403:sgl)
                          n109 = Multiply(x=w402, y=w403) -> (x*y=→"Uref (m/s)":sgl)
                          n110 = call "Calc Force vector.vi"("Pdyn ref (Pa)"=w400, "Cp distribution (time averaged)"=w401) -> ("Fy (N)"=w397:sgl, "Fx (N)"=w398:sgl)
                          "Fx (N)" <- w398
                          "Fy (N)" <- w397
                          n111 = case shown="True" "Snapshot" {
                            tunnel: "Filename (full path)" -> [_ w434]
                            tunnel: w401 -> [_ w433]
                            tunnel: w411 -> [_ w432]
                            tunnel: [errorcluster {"status"=FALSE, "code"=0, "source"=""} ("error out") w429] -> w410
                            tunnel: w400 -> [_ w430]
                            tunnel: w399 -> [_ w428]
                            tunnel: w398 -> [_ w427]
                            tunnel: w397 -> [_ w426]
                            frame False {
                              n112 = local write "ok"(FALSE ("ok")) -> ()
                            }
                            frame True {
                              n113 = local write "Snapshot"(FALSE ("Snapshot")) -> ()
                              n114 = call "Save Cp snapshot.vi"("Pdyn ref (Pa)"=w430, "rho ref (kg/m^3)"=w428, "Fx (N)"=w427, "Fy (N)"=w426, "Cp distribution (time averaged)"=w433, "d.p"=w432, "File Path"=w434) -> ("error out"=w429:errorcluster)  [unwired: 12 in]
                              n115 = Unbundle(w429) -> ("status"=w425:bool)  [unwired: 2 out]
                              n116 = Not(x=w425) -> (.not. x?=→"ok":bool)
                            }
                          }
                        }
                      }
                      n117 = Merge Errors(w315, w314) -> (w313:errorcluster)
                    }
                    frame 1 {
                      n118 = call "Process Data Buffer, Mode 1.vi"("DATA_Buffer excluding '#' [1...N]"=w471, "P constants"=w470) -> ("Pressures (Pa)"=w452:sgl[], "Sensor temps (degC)"=w444:sgl[], "Statuses"=w446:u8[], "dt_warn"=w468:u8)
                      n119 = case shown="True" w442 {
                        tunnel: w468 -> [_ w499]
                        tunnel: w467 -> [_ w498]
                        tunnel: w466 -> [w478 w496]
                        tunnel: w465 -> [w479 w495]
                        tunnel: [w480 w494] -> w464
                        tunnel: w463 -> [_ w493]
                        tunnel: w462 -> [_ w490]
                        tunnel: w461 -> [w480 w489]
                        tunnel: w459 -> [w477 w488]
                        tunnel: [w477 w487] -> w458
                        tunnel: [w479 w486] -> w436
                        tunnel: [w478 w485] -> w457
                        tunnel: w452 -> [w475 w483]
                        tunnel: w446 -> [w474 w482]
                        tunnel: w444 -> [w476 w484]
                        tunnel: [w476 w484] -> w441
                        tunnel: [w475 w483] -> w439
                        tunnel: [w474 w482] -> w440
                        tunnel: [w473 w481] -> w438
                        frame False {
                          n120 = Tick Count (ms)() -> (millisecond timer value=w473:u32)
                        }
                        frame True {
                          # "write after interval has passed, else append. Only if saving data"
                          n121 = Tick Count (ms)() -> (millisecond timer value=w481:u32)
                          n122 = Bundle By Name(cluster=T9 {"Time Stamp"=timestamp(3537581686.1176577 s since 1904-01-01), "dt (us)"=0.0, "dt_warn"=0, "Pressures"=[], "Die temps."=[], "Statuses"=[]} ("P data (Mode 1)"), "Time Stamp"=w498, "dt (us)"=w493, "dt_warn"=w499, "Pressures"=w483, "Statuses"=w482, "Die temps."=w484) -> (w497:T9)
                          n123 = Subtract(x=w481, y=w489) -> (x-y=w492:u32)
                          n124 = Greater Or Equal?(x=w492, y=w490) -> (x >= y?=w491:bool)
                          n125 = case shown="True" w491 {
                            tunnel: [w502 w515] -> w486
                            tunnel: w495 -> [w502 w514]
                            tunnel: w496 -> [w503 w513]
                            tunnel: [w503 w512] -> w485
                            tunnel: w497 -> [w505 w511]
                            tunnel: w488 -> [w506 w510]
                            tunnel: [w504 T9[] []] -> w487
                            tunnel: w481 -> [_ w509]
                            tunnel: [w501 w509] -> w494
                            tunnel: w489 -> [w501 _]
                            frame False {
                              n126 = Build Array (concatenate)(w506, w505) -> (w504:T9[])
                            }
                            frame True {
                              n127 = Build Array (concatenate)(w510, w511) -> (w508:T9[])
                              n128 = call "Datalog append DATA, Mode 1.vi"("Datalog (Data) path"=w513, "Data (Mode 1)"=w508, "Error in"=w514) -> ("Path out"=w512:path, "Error out"=w515:errorcluster)  [unwired: 5 in]
                            }
                          }
                        }
                      }
                      n129 = Subtract(x=w438, y=w447) -> (x-y=w450:u32)
                      n130 = Greater Or Equal?(x=w450, y=w448) -> (x >= y?=w449:bool)
                      n131 = Type Cast(type=FALSE ("Clock drift"), x=w468) -> (*(type *) &x=w460:bool)
                      n132 = case shown="True" w449 {
                        tunnel: [w526 w555] -> w451
                        tunnel: w447 -> [w526 _]
                        tunnel: w438 -> [_ w555]
                        tunnel: w439 -> [w525 w553]
                        tunnel: [w524 sgl[][] []] -> w455
                        tunnel: w453 -> [w523 w554]
                        tunnel: w440 -> [w522 w550]
                        tunnel: [w521 u8[][] []] -> w456
                        tunnel: w454 -> [w520 w551]
                        tunnel: [w519 sgl[][] []] -> w445
                        tunnel: w441 -> [w518 w546]
                        tunnel: w443 -> [w517 w547]
                        tunnel: [errorcluster {"status"=FALSE, "code"=0, "source"=""} ("error out") w542] -> w435
                        frame False {
                          n133 = Build Array (concatenate)(w520, w522) -> (w521:u8[][])
                          n134 = Build Array (concatenate)(w523, w525) -> (w524:sgl[][])
                          n135 = Build Array (concatenate)(w517, w518) -> (w519:sgl[][])
                        }
                        frame True {
                          n136 = Build Array (concatenate)(w551, w550) -> (w544:u8[][])
                          n137 = Build Array (concatenate)(w554, w553) -> (w543:sgl[][])
                          n138 = Build Array (concatenate)(w547, w546) -> (→"Sensor temperatures time trace (Mode \"P & T\" only)":sgl[][])
                          n139 = local write "Stale samples flag"(w544) -> ()
                          n140 = local read "Environmental state values"() -> (w536:T4)
                          n141 = Unbundle By Name(w536) -> ("Density (kg/m^3)"=w529:sgl)
                          n142 = local write "Pressures time trace"(w543) -> ()
                          n143 = local read "Filename (full path)"() -> (w541:path)
                          n144 = call "Create Cp plot.vi"("Pressures in (cols = sensor, rows = time)"=w543) -> ("Cp against x/c"=w531:cluster{"x/c flap (sorted)":sgl[], sgl[]}[], "Pdyn ref (Pa)"=w530:sgl)
                          n145 = local write "Cp distribution (time averaged)"(w531) -> ()
                          n146 = Sign(1:w530) -> (0:w533:sgl)
                          n147 = Add(x=w530, y=w530) -> (x+y=w538:sgl)
                          n148 = local read "Snapshot"() -> (w539:bool)
                          n149 = Absolute Value(x=w538) -> (abs(x)=w532:sgl)
                          n150 = local read "d.p"() -> (w540:i16)
                          n151 = Divide(x=w532, y=w529) -> (x/y=w537:sgl)
                          n152 = Square Root(x=w537) -> (sqrt(x)=w535:sgl)
                          n153 = Multiply(x=w533, y=w535) -> (x*y=w534:sgl)
                          n154 = call "Calc Force vector.vi"("Pdyn ref (Pa)"=w530, "Cp distribution (time averaged)"=w531) -> ("Fy (N)"=w527:sgl, "Fx (N)"=w528:sgl)
                          n155 = case shown="True" w539 {
                            tunnel: w541 -> [_ w567]
                            tunnel: w531 -> [_ w565]
                            tunnel: w540 -> [_ w566]
                            tunnel: [errorcluster {"status"=FALSE, "code"=0, "source"=""} ("error out") w560] -> w542
                            tunnel: w530 -> [_ w564]
                            tunnel: w529 -> [_ w563]
                            tunnel: w528 -> [_ w562]
                            tunnel: w527 -> [_ w561]
                            frame False {
                              n156 = local write "ok"(FALSE ("ok")) -> ()
                            }
                            frame True {
                              n157 = local write "Snapshot"(FALSE ("Snapshot")) -> ()
                              n158 = call "Save Cp snapshot.vi"("Pdyn ref (Pa)"=w564, "rho ref (kg/m^3)"=w563, "Fx (N)"=w562, "Fy (N)"=w561, "Cp distribution (time averaged)"=w565, "d.p"=w566, "File Path"=w567) -> ("error out"=w560:errorcluster)  [unwired: 12 in]
                              n159 = Unbundle(w560) -> ("status"=w559:bool)  [unwired: 2 out]
                              n160 = Not(x=w559) -> (.not. x?=w558:bool)
                              n161 = local write "ok"(w558) -> ()
                            }
                          }
                          n162 = local write "Uref (m/s)"(w534) -> ()
                          n163 = local write "Fx (N)"(w528) -> ()
                          n164 = local write "Fy (N)"(w527) -> ()
                        }
                      }
                      n165 = Merge Errors(w436, w435) -> (w437:errorcluster)
                    }
                  }
                  n166 = Increment(x=w276) -> (x+1=w277:u32)
                  "Samples acquired" <- w276
                }
                frame "$" {
                  n167 = local read "AccelGyro constants"() -> (w593:T2)
                  n168 = VISA Read(VISA resource name=w598, byte count=u32 29, error in (no error)=w597) -> (VISA resource name out=w595:refnum<visa-resource-name>, read buffer=w594:string, error out=w596:errorcluster)  [unwired: 1 out]
                  n169 = call "Process State Buffer.vi"("AccelGyro constants"=w593, "STATE_Buffer excluding '$' [1...30]"=w594) -> ("Inertial state values"=w581:T3, "Environmental state values"=w582:T4)
                  "Environmental state values" <- w582
                  "Inertial state values" <- w581
                  n170 = case shown="True" w589 {
                    tunnel: w582 -> [_ w620]
                    tunnel: w581 -> [_ w619]
                    tunnel: w592 -> [_ w618]
                    tunnel: [w603 w617] -> w591
                    tunnel: w590 -> [w603 w616]
                    tunnel: w588 -> [w602 w615]
                    tunnel: [w602 w614] -> w587
                    tunnel: [w601 w612] -> w586
                    tunnel: w585 -> [w601 w611]
                    tunnel: w584 -> [_ w609]
                    tunnel: [w600 w606] -> w583
                    tunnel: w579 -> [w600 w605]
                    tunnel: w575 -> [_ w604]
                    frame False {
                    }
                    frame True {
                      # "write after interval has passed, else append"
                      n171 = Tick Count (ms)() -> (millisecond timer value=w608:u32)
                      n172 = Subtract(x=w608, y=w605) -> (x-y=w610:u32)
                      n173 = Bundle By Name(cluster=T8 {"Time Stamp"=timestamp(0 s since 1904-01-01), "dt (ms)"=0, "Environmental state values"={"Thermistor (degC)"=0.0, "Sensor temp. (degC)"=0.0, "P_atmos (Pa)"=0.0, "Rel. Humidity (%)"=0.0, "Density (kg/m^3)"=0.0, "Dew point (degC)"=0.0, "Pressure alt. (m)"=0.0, "Density alt. (m)"=0.0}, "Inertial state values"={"w_x (dps)"=0.0, "w_y (dps)"=0.0, "w_z (dps)"=0.0, "a_x (g)"=0.0, "a_y (g)"=0.0, "a_z (g)"=0.0, "Stale sample"=0, "Sensor temp. (degC)"=0.0}} ("All state values"), "Time Stamp"=w618, "dt (ms)"=w604, "Environmental state values"=w620, "Inertial state values"=w619) -> (w613:T8)
                      n174 = Greater Or Equal?(x=w610, y=w609) -> (x >= y?=w607:bool)
                      n175 = case shown="True" w607 {
                        tunnel: [w623 w636] -> w617
                        tunnel: w616 -> [w623 w635]
                        tunnel: w615 -> [w624 w634]
                        tunnel: [w624 w633] -> w614
                        tunnel: w613 -> [w626 w632]
                        tunnel: w611 -> [w627 w631]
                        tunnel: [w625 T8[] []] -> w612
                        tunnel: w608 -> [_ w628]
                        tunnel: [w622 w628] -> w606
                        tunnel: w605 -> [w622 _]
                        frame False {
                          n176 = Build Array (concatenate)(w627, w626) -> (w625:T8[])
                        }
                        frame True {
                          n177 = Build Array (concatenate)(w631, w632) -> (w630:T8[])
                          n178 = call "Datalog append STATE.vi"("Datalog (State) path"=w634, "All state values"=w630, "Error in"=w635) -> ("Path out"=w633:path, "Error out"=w636:errorcluster)  [unwired: 5 in]
                        }
                      }
                    }
                  }
                }
                frame Default {
                }
              }
              "Clock drift" <- w239
              n179 = Or(x="Stop streaming", y=w260) -> (x .or. y?=w259:bool)
            }
            n180 = local read "Data rate (Hz)"() -> (w153:dbl)
            n181 = Reciprocal(x=w153) -> (1/x=w152:dbl)
            n182 = property on="Pressures time trace" class="WFChart (strict)"("XScale.Multiplier"=w152) -> ()  [unwired: 2 in, 2 out]
            n183 = property on="Sensor temperatures time trace (Mode \"P & T\" only)" class="WFChart (strict)"("XScale.Multiplier"=w152) -> ()  [unwired: 2 in, 2 out]
            n184 = call "Stop data stream (s).vi"("VISA resource name in"=w189, "Error In"=w190) -> ("VISA resource name out"=w187:refnum<visa-resource-name>, "Error out"=w188:errorcluster)  [unwired: 7 in]
            n185 = call "Clear buffer.vi"("Error in"=w188, "dt for timeout (ms)"=w185, "VISA resource name in"=w187) -> ("Error out"=w133:errorcluster, "VISA resource name out"=w134:refnum<visa-resource-name>)  [unwired: 3 in]
            n186 = case shown="True" "Save data" {
              tunnel: w143 -> [_ w207]
              tunnel: w142 -> [w198 w206]
              tunnel: w141 -> [_ w205]
              tunnel: w140 -> [_ w204]
              tunnel: w139 -> [_ w203]
              tunnel: w138 -> [_ w202]
              tunnel: [w198 w200] -> w137
              tunnel: w136 -> [_ w199]
              frame False {
              }
              frame True {
                n187 = case shown="0, Default" w204 {
                  tunnel: w207 -> [_ w215]
                  tunnel: w206 -> [w211 w214]
                  tunnel: [w210 w213] -> w201
                  tunnel: w205 -> [w208 w212]
                  tunnel: w203 -> [w209 _]
                  frame 0, Default {
                    n188 = call "Datalog append DATA, Mode 0.vi"("Datalog (Data) path"=w208, "Data (Mode 0)"=w209, "Error in"=w211) -> ("Error out"=w210:errorcluster)  [unwired: 5 in, 1 out]
                  }
                  frame 1 {
                    n189 = call "Datalog append DATA, Mode 1.vi"("Datalog (Data) path"=w212, "Data (Mode 1)"=w215, "Error in"=w214) -> ("Error out"=w213:errorcluster)  [unwired: 5 in, 1 out]
                  }
                }
                n190 = call "Datalog append STATE.vi"("Datalog (State) path"=w199, "All state values"=w202, "Error in"=w201) -> ("Error out"=w200:errorcluster)  [unwired: 5 in, 1 out]
              }
            }
            n191 = call "Close serial port.vi"("Error in"=w133, "VISA resource name"=w134) -> ("Error out"=w184:errorcluster)  [unwired: 9 in]
            n192 = Merge Errors(w184, w137) -> (w183:errorcluster)
          }
        }
        n193 = Dequeue Element(queue=w125, error in (no error)=w124) -> (error out=w123:errorcluster)  [unwired: 1 in, 3 out]
      }
      frame "T" {
        # "dequeue \"busy\" status"
        n194 = Enqueue Element At Opposite End(queue=w664, element=T7 "Busy" ("Cmd"), error in (no error)=w663) -> (queue out=w662:refnum<queue>, error out=w661:errorcluster)  [unwired: 1 in, 1 out]
        n195 = flat-sequence {
          tunnel: w662 -> [w677]
          tunnel: w661 -> [w676]
          tunnel: [w677] -> w660
          tunnel: [w676] -> w659
          tunnel: [TRUE] -> w657
          tunnel: [w670] -> w656
          frame #0 {
            n196 = local read "Serial port"() -> (w669:refnum<visa-resource-name>)
            n197 = Divide(x=1000000.0, y="Data rate (Hz)") -> (x/y=w667:dbl)
            n198 = call "Open serial port.vi"("VISA resource name"=w669) -> ("Error out"=w673:errorcluster, "VISA resource name out"=w674:refnum<visa-resource-name>)  [unwired: 9 in]
            n199 = call "Set stream dt (T).vi"("Error In"=w673, "dt (us)"=w667, "VISA resource name in"=w674) -> ("Error out"=w672:errorcluster, "ACK"=→"ACK 2":bool, "VISA resource name out"=w671:refnum<visa-resource-name>)  [unwired: 6 in]
            n200 = call "Close serial port.vi"("Error in"=w672, "VISA resource name"=w671) -> ("Error out"=w670:errorcluster)  [unwired: 9 in]
          }
        }
        n201 = Dequeue Element(queue=w660, error in (no error)=w659) -> (error out=w658:errorcluster)  [unwired: 1 in, 3 out]
      }
      frame "t" {
        # "dequeue \"busy\" status"
        n202 = Enqueue Element At Opposite End(queue=w689, element=T7 "Busy" ("Cmd"), error in (no error)=w688) -> (queue out=w687:refnum<queue>, error out=w686:errorcluster)  [unwired: 1 in, 1 out]
        n203 = flat-sequence {
          tunnel: w687 -> [w701]
          tunnel: w686 -> [w700]
          tunnel: [w701] -> w685
          tunnel: [w700] -> w684
          tunnel: [TRUE] -> w682
          tunnel: [w694] -> w681
          frame #0 {
            n204 = local read "Env. period (ms)"() -> (w691:i32)
            n205 = local read "Serial port"() -> (w692:refnum<visa-resource-name>)
            n206 = To Unsigned Long Integer(number=w691) -> (unsigned 32bit integer=w690:u32)
            n207 = call "Open serial port.vi"("VISA resource name"=w692) -> ("Error out"=w697:errorcluster, "VISA resource name out"=w698:refnum<visa-resource-name>)  [unwired: 9 in]
            n208 = call "Set state dt (t).vi"("Error In"=w697, "dt (ms)"=w690, "VISA resource name in"=w698) -> ("Error out"=w696:errorcluster, "ACK"=w693:bool, "VISA resource name out"=w695:refnum<visa-resource-name>)  [unwired: 6 in]
            n209 = call "Close serial port.vi"("Error in"=w696, "VISA resource name"=w695) -> ("Error out"=w694:errorcluster)  [unwired: 9 in]
            n210 = local write "ACK 2"(w693) -> ()
          }
        }
        n211 = Dequeue Element(queue=w685, error in (no error)=w684) -> (error out=w683:errorcluster)  [unwired: 1 in, 3 out]
      }
      frame "M" {
        # "dequeue \"busy\" status"
        n212 = Enqueue Element At Opposite End(queue=w713, element=T7 "Busy" ("Cmd"), error in (no error)=w712) -> (queue out=w711:refnum<queue>, error out=w710:errorcluster)  [unwired: 1 in, 1 out]
        n213 = flat-sequence {
          tunnel: w711 -> [w725]
          tunnel: w710 -> [w724]
          tunnel: [w725] -> w709
          tunnel: [w724] -> w708
          tunnel: [TRUE] -> w706
          tunnel: [w718] -> w705
          frame #0 {
            n214 = local read "Serial port"() -> (w716:refnum<visa-resource-name>)
            n215 = call "Open serial port.vi"("VISA resource name"=w716) -> ("Error out"=w721:errorcluster, "VISA resource name out"=w722:refnum<visa-resource-name>)  [unwired: 9 in]
            n216 = call "Set mode (M).vi"("Error In"=w721, "Mode"="Data mode", "VISA resource name in"=w722) -> ("Error out"=w720:errorcluster, "ACK"=w717:bool, "L_data"=→"L_data (bytes)":u16, "VISA resource name out"=w719:refnum<visa-resource-name>)  [unwired: 5 in]
            n217 = call "Close serial port.vi"("Error in"=w720, "VISA resource name"=w719) -> ("Error out"=w718:errorcluster)  [unwired: 9 in]
            n218 = local write "ACK 2"(w717) -> ()
          }
        }
        n219 = Dequeue Element(queue=w709, error in (no error)=w708) -> (error out=w707:errorcluster)  [unwired: 1 in, 3 out]
      }
      frame "O" {
        # "dequeue \"busy\" status"
        n220 = Enqueue Element At Opposite End(queue=w737, element=T7 "Busy" ("Cmd"), error in (no error)=w736) -> (queue out=w735:refnum<queue>, error out=w734:errorcluster)  [unwired: 1 in, 1 out]
        n221 = flat-sequence {
          tunnel: w735 -> [w749]
          tunnel: w734 -> [w748]
          tunnel: [w749] -> w733
          tunnel: [w748] -> w732
          tunnel: [TRUE] -> w730
          tunnel: [w742] -> w729
          frame #0 {
            n222 = local read "Serial port"() -> (w741:refnum<visa-resource-name>)
            n223 = call "Open serial port.vi"("VISA resource name"=w741) -> ("Error out"=w745:errorcluster, "VISA resource name out"=w746:refnum<visa-resource-name>)  [unwired: 9 in]
            n224 = call "Override maxSensorNum (O).vi"("Error In"=w745, "Max. number of sensors"="Max. num. sensors (override)", "VISA resource name in"=w746) -> ("Error out"=w744:errorcluster, "ACK"=→"ACK 3":bool, "L_data"=w738:u16, "VISA resource name out"=w743:refnum<visa-resource-name>)  [unwired: 5 in]
            n225 = local write "L_data (bytes)"(w738) -> ()
            n226 = call "Close serial port.vi"("Error in"=w744, "VISA resource name"=w743) -> ("Error out"=w742:errorcluster)  [unwired: 9 in]
          }
        }
        n227 = Dequeue Element(queue=w733, error in (no error)=w732) -> (error out=w731:errorcluster)  [unwired: 1 in, 3 out]
      }
      frame "G" {
        # "dequeue \"busy\" status"
        n228 = Enqueue Element At Opposite End(queue=w761, element=T7 "Busy" ("Cmd"), error in (no error)=w760) -> (queue out=w759:refnum<queue>, error out=w758:errorcluster)  [unwired: 1 in, 1 out]
        n229 = flat-sequence {
          tunnel: w759 -> [w777]
          tunnel: w758 -> [w776]
          tunnel: [w777] -> w757
          tunnel: [w776] -> w756
          tunnel: [TRUE] -> w754
          tunnel: [w770] -> w753
          frame #0 {
            n230 = local read "Serial port"() -> (w769:refnum<visa-resource-name>)
            n231 = call "Open serial port.vi"("VISA resource name"=w769) -> ("Error out"=w773:errorcluster, "VISA resource name out"=w774:refnum<visa-resource-name>)  [unwired: 9 in]
            n232 = call "Get status bits 1 (G).vi"("VISA resource name in"=w774, "Error In"=w773) -> ("nFaults"=w766:u8, "nSensors"=w765:u8, "nCards"=w764:u8, "PowerState"=w763:bool, "VISA resource name out"=w771:refnum<visa-resource-name>, "ACK"=→"ACK 5":bool, "Error out"=w772:errorcluster)  [unwired: 11 in]
            n233 = local read "System status"() -> (w762:T5)
            n234 = call "Close serial port.vi"("Error in"=w772, "VISA resource name"=w771) -> ("Error out"=w770:errorcluster)  [unwired: 9 in]
            n235 = Bundle By Name(cluster=w762, "Main power"=w763, "Occupied slots"=w764, "Active sensors"=w765, "Faulty sensors"=w766) -> (→"System status":T5)
          }
        }
        n236 = Dequeue Element(queue=w757, error in (no error)=w756) -> (error out=w755:errorcluster)  [unwired: 1 in, 3 out]
      }
      frame "g" {
        # "dequeue \"busy\" status"
        n237 = Enqueue Element At Opposite End(queue=w789, element=T7 "Busy" ("Cmd"), error in (no error)=w788) -> (queue out=w787:refnum<queue>, error out=w786:errorcluster)  [unwired: 1 in, 1 out]
        n238 = flat-sequence {
          tunnel: w787 -> [w810]
          tunnel: w786 -> [w809]
          tunnel: [w810] -> w785
          tunnel: [w809] -> w784
          tunnel: [TRUE] -> w782
          tunnel: [w803] -> w781
          frame #0 {
            w792 = T11."Disabled and Grayed Out" ("Disabled")
            w791 = T11."Enabled" ("Disabled")
            n239 = local read "Serial port"() -> (w802:refnum<visa-resource-name>)
            n240 = call "Open serial port.vi"("VISA resource name"=w802) -> ("Error out"=w806:errorcluster, "VISA resource name out"=w807:refnum<visa-resource-name>)  [unwired: 9 in]
            n241 = call "Get status bits 2 (g).vi"("VISA resource name in"=w807, "Error In"=w806) -> ("Mode"=w801:u8, "Therm_ok"=w793:bool, "BMI160_ok"=w797:bool, "BME280_ok"=w795:bool, "VISA resource name out"=w804:refnum<visa-resource-name>, "ACK"=w799:bool, "Error out"=w805:errorcluster)  [unwired: 11 in]
            n242 = Select(t=w791, s=w793, f=w792) -> (s? t:f=w796:T11)
            n243 = Select(t=w791, s=w795, f=w792) -> (s? t:f=w794:T11)
            n244 = stacked-sequence {
              tunnel: w796 -> [_ w812]
              tunnel: w794 -> [w811 _]
              tunnel: w793 -> [_ w813]
              frame #0 {
                n245 = property on="Environmental state values" class="Clust (strict)"("DisabledEnum"=w811) -> ()  [unwired: 2 in, 2 out]
                n246 = property on="Density (kg/m^3)" class="DigNum (strict)"("DisabledEnum"=w811) -> ()  [unwired: 2 in, 2 out]
                n247 = property on="Dew point (degC)" class="DigNum (strict)"("DisabledEnum"=w811) -> ()  [unwired: 2 in, 2 out]
                n248 = property on="Density alt. (m)" class="DigNum (strict)"("DisabledEnum"=w811) -> ()  [unwired: 2 in, 2 out]
              }
              frame #1 {
                n249 = case shown="False" w813 {
                  tunnel: w812 -> [w814 _]
                  frame False {
                    n250 = property on="Density (kg/m^3)" class="DigNum (strict)"("DisabledEnum"=w814) -> ()  [unwired: 2 in, 2 out]
                    n251 = property on="Dew point (degC)" class="DigNum (strict)"("DisabledEnum"=w814) -> ()  [unwired: 2 in, 2 out]
                    n252 = property on="Density alt. (m)" class="DigNum (strict)"("DisabledEnum"=w814) -> ()  [unwired: 2 in, 2 out]
                  }
                  frame True {
                  }
                }
                n253 = property on="Thermistor (degC)" class="DigNum (strict)"("DisabledEnum"=w812) -> ()  [unwired: 2 in, 2 out]
              }
            }
            n254 = local read "System status"() -> (w798:T5)
            n255 = call "Close serial port.vi"("Error in"=w805, "VISA resource name"=w804) -> ("Error out"=w803:errorcluster)  [unwired: 9 in]
            n256 = local write "ACK 5"(w799) -> ()
            n257 = Select(t=w791, s=w797, f=w792) -> (s? t:f=w790:T11)
            n258 = Bundle By Name(cluster=w798, "Env. sensor"=w795, "Inertial sensor"=w797, "Thermistor"=w793, "Mode"=w801) -> (w800:T5)
            n259 = property on="Inertial state values" class="Clust (strict)"("DisabledEnum"=w790) -> ()  [unwired: 2 in, 2 out]
            n260 = property on="AccelGyro constants" class="Clust (strict)"("DisabledEnum"=w790) -> ()  [unwired: 2 in, 2 out]
            n261 = property on="Accel. range (g)" class="Ring (strict)"("DisabledEnum"=w790) -> ()  [unwired: 2 in, 2 out]
            n262 = property on="Accel. rate (Hz)" class="Ring (strict)"("DisabledEnum"=w790) -> ()  [unwired: 2 in, 2 out]
            n263 = property on="Gyro. range (dps)" class="Ring (strict)"("DisabledEnum"=w790) -> ()  [unwired: 2 in, 2 out]
            n264 = property on="Gyro. rate (Hz)" class="Ring (strict)"("DisabledEnum"=w790) -> ()  [unwired: 2 in, 2 out]
            n265 = property on="Apply settings 3" class="Bool"("DisabledEnum"=w790) -> ()  [unwired: 2 in, 2 out]
            n266 = property on="ACK 8" class="Bool (strict)"("DisabledEnum"=w790) -> ()  [unwired: 2 in, 2 out]
            n267 = local write "System status"(w800) -> ()
          }
        }
        n268 = Dequeue Element(queue=w785, error in (no error)=w784) -> (error out=w783:errorcluster)  [unwired: 1 in, 3 out]
      }
      frame "F" {
        # "dequeue \"busy\" status"
        n269 = Enqueue Element At Opposite End(queue=w826, element=T7 "Busy" ("Cmd"), error in (no error)=w825) -> (queue out=w824:refnum<queue>, error out=w823:errorcluster)  [unwired: 1 in, 1 out]
        n270 = flat-sequence {
          tunnel: w824 -> [w836]
          tunnel: w823 -> [w835]
          tunnel: [w836] -> w822
          tunnel: [w835] -> w821
          tunnel: [TRUE] -> w819
          tunnel: [w829] -> w818
          frame #0 {
            n271 = local read "Serial port"() -> (w828:refnum<visa-resource-name>)
            n272 = call "Open serial port.vi"("VISA resource name"=w828) -> ("Error out"=w832:errorcluster, "VISA resource name out"=w833:refnum<visa-resource-name>)  [unwired: 9 in]
            n273 = call "Collate faulty sensor indices.vi"("Error In"=w832, "VISA resource name in"=w833) -> ("Error out"=w831:errorcluster, "Faulty sensor indices"=→"Faulty sensors":i32[], "VISA resource name out"=w830:refnum<visa-resource-name>)  [unwired: 7 in]
            n274 = call "Close serial port.vi"("Error in"=w831, "VISA resource name"=w830) -> ("Error out"=w829:errorcluster)  [unwired: 9 in]
          }
        }
        n275 = Dequeue Element(queue=w822, error in (no error)=w821) -> (error out=w820:errorcluster)  [unwired: 1 in, 3 out]
      }
      frame "A" {
        # "dequeue \"busy\" status"
        n276 = Enqueue Element At Opposite End(queue=w848, element=T7 "Busy" ("Cmd"), error in (no error)=w847) -> (queue out=w846:refnum<queue>, error out=w845:errorcluster)  [unwired: 1 in, 1 out]
        n277 = flat-sequence {
          tunnel: w846 -> [w858]
          tunnel: w845 -> [w857]
          tunnel: [w858] -> w844
          tunnel: [w857] -> w843
          tunnel: [TRUE] -> w841
          tunnel: [w851] -> w840
          frame #0 {
            n278 = local read "Serial port"() -> (w850:refnum<visa-resource-name>)
            n279 = call "Open serial port.vi"("VISA resource name"=w850) -> ("Error out"=w854:errorcluster, "VISA resource name out"=w855:refnum<visa-resource-name>)  [unwired: 9 in]
            n280 = call "Collate active sensor indices.vi"("Error In"=w854, "VISA resource name in"=w855) -> ("Error out"=w853:errorcluster, "Active sensor indices"=→"Active sensors":i32[], "VISA resource name out"=w852:refnum<visa-resource-name>)  [unwired: 7 in]
            n281 = call "Close serial port.vi"("Error in"=w853, "VISA resource name"=w852) -> ("Error out"=w851:errorcluster)  [unwired: 9 in]
          }
        }
        n282 = Dequeue Element(queue=w844, error in (no error)=w843) -> (error out=w842:errorcluster)  [unwired: 1 in, 3 out]
      }
      frame "C" {
        # "dequeue \"busy\" status"
        n283 = Enqueue Element At Opposite End(queue=w870, element=T7 "Busy" ("Cmd"), error in (no error)=w869) -> (queue out=w868:refnum<queue>, error out=w867:errorcluster)  [unwired: 1 in, 1 out]
        n284 = flat-sequence {
          tunnel: w868 -> [w888]
          tunnel: w867 -> [w887]
          tunnel: [w888] -> w866
          tunnel: [w887] -> w865
          tunnel: [TRUE] -> w863
          tunnel: [w881] -> w862
          frame #0 {
            n285 = local read "Serial port"() -> (w880:refnum<visa-resource-name>)
            n286 = call "Open serial port.vi"("VISA resource name"=w880) -> ("Error out"=w884:errorcluster, "VISA resource name out"=w885:refnum<visa-resource-name>)  [unwired: 9 in]
            n287 = call "Configure BMI160 (C).vi"("VISA resource name in"=w885, "Accel. range (g)"="Accel. range (g)", "Accel. rate (Hz)"="Accel. rate (Hz)", "Gyro. range (dps)"="Gyro. range (dps)", "Gyro. rate (Hz)"="Gyro. rate (Hz)", "Error In"=w884) -> ("VISA resource name out"=w882:refnum<visa-resource-name>, "ACK ok"=→"ACK 4":bool, "Error out"=w883:errorcluster)  [unwired: 11 in]
            n288 = case shown="0, Default" "Accel. range (g)" {
              tunnel: [sgl 2.0 ("accRange") sgl 4.0 ("accRange") sgl 8.0 ("accRange") sgl 16.0 ("accRange")] -> w874
              frame 0, Default {
              }
              frame 1 {
              }
              frame 2 {
              }
              frame 3 {
              }
            }
            n289 = case shown="0, Default" "Gyro. range (dps)" {
              tunnel: [sgl 125.0 ("accRange") sgl 250.0 ("accRange") sgl 500.0 ("accRange") sgl 1000.0 ("accRange") sgl 2000.0 ("accRange")] -> w872
              frame 0, Default {
              }
              frame 1 {
              }
              frame 2 {
              }
              frame 3 {
              }
              frame 4 {
              }
            }
            n290 = call "Close serial port.vi"("Error in"=w883, "VISA resource name"=w882) -> ("Error out"=w881:errorcluster)  [unwired: 9 in]
            n291 = local read "AccelGyro constants"() -> (w871:T2)
            n292 = Bundle By Name(cluster=w871, "accRange"=w874, "gyrRange"=w872) -> (w876:T2)
            n293 = local write "AccelGyro constants"(w876) -> ()
          }
        }
        n294 = Dequeue Element(queue=w866, error in (no error)=w865) -> (error out=w864:errorcluster)  [unwired: 1 in, 3 out]
      }
      frame "Z" {
        # "dequeue \"busy\" status"
        n295 = Enqueue Element At Opposite End(queue=w909, element=T7 "Busy" ("Cmd"), error in (no error)=w908) -> (queue out=w907:refnum<queue>, error out=w906:errorcluster)  [unwired: 1 in, 1 out]
        n296 = flat-sequence {
          tunnel: w907 -> [w919]
          tunnel: w906 -> [w918]
          tunnel: [w919] -> w905
          tunnel: [w918] -> w904
          tunnel: [TRUE] -> w902
          tunnel: [w912] -> w901
          frame #0 {
            n297 = local read "Serial port"() -> (w911:refnum<visa-resource-name>)
            n298 = call "Open serial port.vi"("VISA resource name"=w911) -> ("Error out"=w915:errorcluster, "VISA resource name out"=w916:refnum<visa-resource-name>)  [unwired: 9 in]
            n299 = call "Get Serial Number (Z).vi"("VISA resource name in"=w916, "Error In"=w915) -> ("VISA resource name out"=w913:refnum<visa-resource-name>, "Serial Number"=→"Serial no.":u16, "Error out"=w914:errorcluster)  [unwired: 5 in, 1 out]
            n300 = call "Close serial port.vi"("Error in"=w914, "VISA resource name"=w913) -> ("Error out"=w912:errorcluster)  [unwired: 9 in]
          }
        }
        n301 = Dequeue Element(queue=w905, error in (no error)=w904) -> (error out=w903:errorcluster)  [unwired: 1 in, 3 out]
      }
      frame "D" {
        # "dequeue \"busy\" status"
        n302 = Enqueue Element At Opposite End(queue=w933, element=T7 "Busy" ("Cmd"), error in (no error)=w932) -> (queue out=w931:refnum<queue>, error out=w930:errorcluster)  [unwired: 1 in, 1 out]
        n303 = flat-sequence {
          tunnel: w931 -> [w956]
          tunnel: w930 -> [w955]
          tunnel: [w956] -> w929
          tunnel: [w955] -> w928
          tunnel: [TRUE] -> w926
          tunnel: [w937] -> w925
          tunnel: [w935] -> w923
          tunnel: w922 -> [w941]
          tunnel: w921 -> [w940]
          tunnel: [w939] -> w920
          frame #0 {
            n304 = local read "Save data"() -> (w936:bool)
            n305 = local read "AccelGyro constants"() -> (w945:T2)
            n306 = local read "Serial port"() -> (w953:refnum<visa-resource-name>)
            n307 = call "Open serial port.vi"("VISA resource name"=w953) -> ("Error out"=w951:errorcluster, "VISA resource name out"=w952:refnum<visa-resource-name>)  [unwired: 9 in]
            n308 = call "Get Env data (oneshot) (D).vi"("VISA resource name in"=w952, "Error In"=w951) -> ("VISA resource name out"=w949:refnum<visa-resource-name>, "STATE_Buffer"=w948:string, "ACK"=→"ACK 6":bool, "Error out"=w950:errorcluster)  [unwired: 5 in]
            n309 = call "Close serial port.vi"("Error in"=w950, "VISA resource name"=w949) -> ("Error out"=w938:errorcluster)  [unwired: 9 in]
            n310 = String Subset(string=w948, offset (0)=1) -> (substring=w947:string)  [unwired: 1 in]
            n311 = call "Process State Buffer.vi"("AccelGyro constants"=w945, "STATE_Buffer excluding '$' [1...30]"=w947) -> ("Inertial state values"=w942:T3, "Environmental state values"=w943:T4)
            n312 = case shown="True" w936 {
              tunnel: w943 -> [_ w980]
              tunnel: w942 -> [_ w979]
              tunnel: [errorcluster {"status"=FALSE, "code"=0, "source"=""} ("Error out") w977] -> w934
              tunnel: [w959 w975] -> w935
              tunnel: w941 -> [w959 w974]
              tunnel: w940 -> [w958 w969]
              tunnel: [w958 w970] -> w939
              frame False {
                (unwired) path "" ("Path out")
              }
              frame True {
                # "write after interval has passed, else append"
                n313 = local read "Datalog name (without extension)"() -> (w962:string)
                n314 = local read "Datalog directory"() -> (w963:path)
                n315 = local read "Write interval (s)"() -> (w967:u32)
                n316 = Concatenate Strings(w962, "_S_.log" ("string")) -> (w964:string)
                n317 = local read "Env. period (ms)"() -> (w978:i32)
                n318 = Get Date/Time In Seconds() -> (seconds since 1Jan1904=w968:timestamp)
                n319 = Build Path(base path=w963, name or relative path=w964) -> (appended path=w961:path)
                n320 = Multiply(x=u32 1000, y=w967) -> (x*y=w966:u32)
                n321 = Tick Count (ms)() -> (millisecond timer value=w972:u32)
                n322 = Subtract(x=w972, y=w969) -> (x-y=w973:u32)
                n323 = Bundle By Name(cluster=T8 {"Time Stamp"=timestamp(0 s since 1904-01-01), "dt (ms)"=0, "Environmental state values"={"Thermistor (degC)"=0.0, "Sensor temp. (degC)"=0.0, "P_atmos (Pa)"=0.0, "Rel. Humidity (%)"=0.0, "Density (kg/m^3)"=0.0, "Dew point (degC)"=0.0, "Pressure alt. (m)"=0.0, "Density alt. (m)"=0.0}, "Inertial state values"={"w_x (dps)"=0.0, "w_y (dps)"=0.0, "w_z (dps)"=0.0, "a_x (g)"=0.0, "a_y (g)"=0.0, "a_z (g)"=0.0, "Stale sample"=0, "Sensor temp. (degC)"=0.0}} ("All state values"), "Time Stamp"=w968, "dt (ms)"=w978, "Environmental state values"=w980, "Inertial state values"=w979) -> (w976:T8)
                n324 = Greater Or Equal?(x=w973, y=w966) -> (x >= y?=w971:bool)
                n325 = case shown="True" w971 {
                  tunnel: [errorcluster {"status"=FALSE, "code"=0, "source"=""} ("Error out") w994] -> w977
                  tunnel: w961 -> [_ w993]
                  tunnel: w976 -> [w985 w992]
                  tunnel: w974 -> [w986 w991]
                  tunnel: [w984 T8[] []] -> w975
                  tunnel: w972 -> [_ w988]
                  tunnel: [w983 w988] -> w970
                  tunnel: w969 -> [w983 _]
                  frame False {
                    n326 = Build Array (concatenate)(w986, w985) -> (w984:T8[])
                  }
                  frame True {
                    n327 = Build Array (concatenate)(w991, w992) -> (w990:T8[])
                    n328 = call "Datalog append STATE.vi"("Datalog (State) path"=w993, "All state values"=w990, "Error in"=errorcluster {"status"=FALSE, "code"=0, "source"=""} ("Error out")) -> ("Error out"=w994:errorcluster)  [unwired: 5 in, 1 out]
                  }
                }
              }
            }
            n329 = local write "Environmental state values"(w943) -> ()
            n330 = local write "Inertial state values"(w942) -> ()
            n331 = Merge Errors(w938, w934) -> (w937:errorcluster)
          }
        }
        n332 = Dequeue Element(queue=w929, error in (no error)=w928) -> (error out=w927:errorcluster)  [unwired: 1 in, 3 out]
      }
      frame "accgyr_consts" {
        # "dequeue \"busy\" status"
        n333 = Enqueue Element At Opposite End(queue=w1006, element=T7 "Busy" ("Cmd"), error in (no error)=w1005) -> (queue out=w1004:refnum<queue>, error out=w1003:errorcluster)  [unwired: 1 in, 1 out]
        n334 = flat-sequence {
          tunnel: w1004 -> [w1026]
          tunnel: w1003 -> [w1025]
          tunnel: [w1026] -> w1002
          tunnel: [w1025] -> w1001
          tunnel: [TRUE] -> w999
          tunnel: [w1023] -> w998
          frame #0 {
            n335 = local read "Serial port"() -> (w1022:refnum<visa-resource-name>)
            n336 = call "Open serial port.vi"("VISA resource name"=w1022) -> ("Error out"=w1020:errorcluster, "VISA resource name out"=w1021:refnum<visa-resource-name>)  [unwired: 9 in]
            n337 = call "Get AccelGyro constants (MCU EEPROM).vi"("VISA resource name in"=w1021, "Error In"=w1020) -> ("VISA resource name out"=w1018:refnum<visa-resource-name>, "AccelGyro constants"=w1015:T2, "ACK"=→"ACK 8":bool, "Error out"=w1019:errorcluster)  [unwired: 5 in]
            n338 = Unbundle By Name(w1015) -> ("gx offset"=w1014:sgl, "gy offset"=w1013:sgl, "gz offset"=w1012:sgl, "ax offset"=w1011:sgl, "ay offset"=w1010:sgl, "az offset"=w1009:sgl, "axyz scale"=w1008:sgl)
            n339 = call "Close serial port.vi"("Error in"=w1019, "VISA resource name"=w1018) -> ("Error out"=w1023:errorcluster)  [unwired: 9 in]
            n340 = Bundle By Name(cluster=T2 {"gyrRange"=125.0, "accRange"=2.0, "gx offset"=0.0, "gy offset"=0.0, "gz offset"=0.0, "ax offset"=0.0, "ay offset"=0.0, "az offset"=0.0, "axyz scale"=1.0} ("AccelGyro constants"), "gx offset"=w1014, "gy offset"=w1013, "gz offset"=w1012, "ax offset"=w1011, "ay offset"=w1010, "az offset"=w1009, "axyz scale"=w1008) -> (→"AccelGyro constants":T2)
          }
        }
        n341 = Dequeue Element(queue=w1002, error in (no error)=w1001) -> (error out=w1000:errorcluster)  [unwired: 1 in, 3 out]
      }
      frame "EEPROM_Pconsts" {
        # "dequeue \"busy\" status"
        n342 = Enqueue Element At Opposite End(queue=w1038, element=T7 "Busy" ("Cmd"), error in (no error)=w1037) -> (queue out=w1036:refnum<queue>, error out=w1035:errorcluster)  [unwired: 1 in, 1 out]
        n343 = flat-sequence {
          tunnel: w1036 -> [w1054]
          tunnel: w1035 -> [w1053]
          tunnel: [w1054] -> w1034
          tunnel: [w1053] -> w1033
          tunnel: [TRUE] -> w1031
          tunnel: [w1051] -> w1030
          frame #0 {
            # "Must only run this case after running \"P\", \"G\", \"A\""
            n344 = local read "System status"() -> (w1043:T5)
            n345 = Unbundle By Name(w1043) -> ("Occupied slots"=w1042:u8)
            n346 = local read "Serial port"() -> (w1050:refnum<visa-resource-name>)
            n347 = To Long Integer(number=w1042) -> (32bit integer=w1041:i32)
            n348 = call "Open serial port.vi"("VISA resource name"=w1050) -> ("Error out"=w1048:errorcluster, "VISA resource name out"=w1049:refnum<visa-resource-name>)  [unwired: 9 in]
            n349 = local read "Active sensors"() -> (w1045:i32[])
            n350 = call "Concatenate all slot EEPROM arrays.vi"("Error In"=w1048, "N slots occupied"=w1041, "VISA resource name in"=w1049) -> ("Error out"=w1047:errorcluster, "ACK (all)"=→"ACK 7":bool, "All slot EEPROM values"=w1040:T12[], "VISA resource name out"=w1046:refnum<visa-resource-name>)  [unwired: 5 in]
            n351 = call "Populate pressure constants array.vi"("Occupied slot EEPROM values"=w1040, "Active sensor indices"=w1045) -> ("Active pressure sensor constants"=→"Active pressure sensor constants":T6[])
            n352 = call "Close serial port.vi"("Error in"=w1047, "VISA resource name"=w1046) -> ("Error out"=w1051:errorcluster)  [unwired: 9 in]
          }
        }
        n353 = Dequeue Element(queue=w1034, error in (no error)=w1033) -> (error out=w1032:errorcluster)  [unwired: 1 in, 3 out]
      }
      frame "convert_datalogs" {
        # "dequeue \"busy\" status"
        n354 = Enqueue Element At Opposite End(queue=w1066, element=T7 "Busy" ("Cmd"), error in (no error)=w1065) -> (queue out=w1064:refnum<queue>, error out=w1063:errorcluster)  [unwired: 1 in, 1 out]
        n355 = flat-sequence {
          tunnel: w1064 -> [w1116]
          tunnel: w1063 -> [w1115]
          tunnel: [w1116] -> w1062
          tunnel: [w1115] -> w1061
          tunnel: [TRUE] -> w1059
          tunnel: [w1095] -> w1058
          frame #0 {
            n356 = local read "System status"() -> (w1106:T5)
            n357 = local read "Datalog name (without extension)"() -> (w1103:string)
            n358 = local read "Datalog name (without extension)"() -> (w1110:string)
            n359 = Unbundle By Name(w1106) -> ("Mode"=w1102:u8)
            n360 = local read "Datalog directory"() -> (w1104:path)
            n361 = local read "Datalog directory"() -> (w1111:path)
            n362 = case shown="0, Default" w1102 {
              tunnel: ["_P0.log" ("string") "_P1.log" ("string")] -> w1105
              frame 0, Default {
              }
              frame 1 {
              }
            }
            n363 = Concatenate Strings(w1103, "_S.log" ("string")) -> (w1107:string)
            n364 = Concatenate Strings(w1110, "_S_.log" ("string")) -> (w1112:string)
            n365 = Concatenate Strings(w1103, w1105) -> (w1109:string)
            n366 = Build Path(base path=w1104, name or relative path=w1109) -> (appended path=w1071:path)
            n367 = Build Path(base path=w1104, name or relative path=w1107) -> (appended path=w1079:path)
            n368 = Build Path(base path=w1111, name or relative path=w1112) -> (appended path=w1093:path)
            n369 = Path To String(path=w1079) -> (string=w1080:string)
            n370 = Path To String(path=w1093) -> (string=w1092:string)
            n371 = Path To String(path=w1071) -> (string=w1077:string)
            n372 = Reverse String(1:w1080) -> (0:w1081:string)
            n373 = Reverse String(1:w1092) -> (0:w1091:string)
            n374 = Reverse String(1:w1077) -> (0:w1076:string)
            n375 = String Subset(string=w1081, offset (0)=3 ("length (rest)")) -> (substring=w1082:string)  [unwired: 1 in]
            n376 = String Subset(string=w1091, offset (0)=3 ("length (rest)")) -> (substring=w1090:string)  [unwired: 1 in]
            n377 = String Subset(string=w1076, offset (0)=3 ("length (rest)")) -> (substring=w1075:string)  [unwired: 1 in]
            n378 = Reverse String(1:w1082) -> (0:w1083:string)
            n379 = Reverse String(1:w1090) -> (0:w1089:string)
            n380 = Reverse String(1:w1075) -> (0:w1074:string)
            n381 = Concatenate Strings(w1083, "txt" ("string")) -> (w1085:string)
            n382 = Concatenate Strings(w1089, "txt" ("string")) -> (w1087:string)
            n383 = Concatenate Strings(w1074, "txt" ("string")) -> (w1072:string)
            n384 = String To Path(string=w1085) -> (path=w1078:path)
            n385 = String To Path(string=w1087) -> (path=w1086:path)
            n386 = String To Path(string=w1072) -> (path=w1070:path)
            n387 = case shown="0, Default" w1102 {
              tunnel: w1071 -> [w1123 w1127]
              tunnel: [w1121 w1125] -> w1098
              tunnel: "d.p" -> [w1120 w1128]
              tunnel: w1070 -> [w1119 w1124]
              frame 0, Default {
                n388 = call "Datalog to ASCII (DATA, Mode 0).vi"("Error in"=errorcluster {"status"=FALSE, "code"=0, "source"=""}, "ASCII output path"=w1119, "Precision"=w1120, "Datalog path"=w1123) -> ("Error out"=w1121:errorcluster)  [unwired: 3 in]
              }
              frame 1 {
                n389 = call "Datalog to ASCII (DATA, Mode 1).vi"("Error in"=errorcluster {"status"=FALSE, "code"=0, "source"=""}, "ASCII output path"=w1124, "Precision"=w1128, "Datalog path"=w1127) -> ("Error out"=w1125:errorcluster)  [unwired: 3 in]
              }
            }
            n390 = call "Datalog to ASCII (STATE).vi"("Error in"=errorcluster {"status"=FALSE, "code"=0, "source"=""}, "ASCII output path"=w1078, "Precision"="d.p", "Datalog path"=w1079) -> ("Error out"=w1097:errorcluster)  [unwired: 3 in]
            n391 = call "Datalog to ASCII (STATE_).vi"("Error in"=errorcluster {"status"=FALSE, "code"=0, "source"=""}, "ASCII output path"=w1086, "Precision"="d.p", "Datalog path"=w1093) -> ("Error out"=w1096:errorcluster)  [unwired: 3 in]
            n392 = Merge Errors(w1098, w1097, w1096) -> (w1095:errorcluster)
            n393 = case shown="No Error" w1095 {
              tunnel: [TRUE FALSE] -> w1094
              frame No Error {
              }
              frame Error {
              }
            }
            "ASCII done" <- w1094
          }
        }
        n394 = Dequeue Element(queue=w1062, error in (no error)=w1061) -> (error out=w1060:errorcluster)  [unwired: 1 in, 3 out]
      }
      frame "Exit", Default {
      }
    }
    n395 = call <vilib>:"Clear Errors.vi"("error in (no error)"=w39, "specific error code to clear (0: all)"=1073676294) -> ("error out"=w38:errorcluster)  [unwired: 4 in, 1 out]
    "Error" <- w38
  }
  n396 = while {
    tunnel: w10 -> [w1140]
    tunnel: w9 -> [w1139]
    tunnel: [w1138] -> w32
    tunnel: [w1137] -> w31
    stop <- w1141 continue-if-true
    n397 = event shown="[0] Timeout" {
      selector: _ -> [_ _ _ _ _ _ _ _ _ _]
      dyn-events: _ -> [_ _ _ _ _ _ _ _ _ _]
      timeout: "Env. period (ms)" -> [_ _ _ _ _ _ _ _ _ _]
      tunnel: [TRUE TRUE w1233 TRUE TRUE TRUE TRUE TRUE TRUE TRUE] -> w1141
      tunnel: w1140 -> [w1154 w1172 w1237 w1265 w1320 w1338 w1366 w1400 w1422 w1441]
      tunnel: w1139 -> [w1153 w1171 w1238 w1264 w1317 w1337 w1365 w1399 w1421 w1440]
      tunnel: [w1151 w1167 w1242 w1263 w1318 w1335 w1364 w1397 w1420 w1438] -> w1138
      tunnel: [w1152 w1168 w1243 w1262 w1319 w1334 w1363 w1398 w1419 w1439] -> w1137
      event Timeout {
        # "only queue msg if not busy"
        n398 = event-data() -> ()  [unwired: 1 in, 1 out]
        n399 = local read "System status"() -> (w1145:T5)
        n400 = Unbundle By Name(w1145) -> ("Main power"=w1144:bool)
        n401 = Preview Queue Element(queue=w1154, timeout in ms (-1)=0, error in (no error)=w1153) -> (queue out=w1148:refnum<queue>, element=w1150:T7, error out=w1147:errorcluster)  [unwired: 1 out]
        n402 = Not Equal?(x=T7 "Busy" ("Cmd"), y=w1150) -> (x != y?=w1143:bool)
        n403 = And(x=w1144, y=w1143) -> (x .and. y?=w1142:bool)
        n404 = case shown="True" w1142 {
          tunnel: w1148 -> [w1157 w1162]
          tunnel: w1147 -> [w1156 w1161]
          tunnel: [w1157 w1159] -> w1152
          tunnel: [w1156 w1160] -> w1151
          frame False {
          }
          frame True {
            n405 = local write "ACK 6"(FALSE ("ACK 6")) -> ()
            n406 = Enqueue Element(queue=w1162, element=T7 "D" ("Cmd"), error in (no error)=w1161) -> (queue out=w1159:refnum<queue>, error out=w1160:errorcluster)  [unwired: 1 in, 1 out]
          }
        }
      }
      event "Main Power": Value Change {
        # "only queue msg if not busy"
        n407 = event-data() -> ("NewVal"=w1164:bool)  [unwired: 1 in, 1 out]
        n408 = Preview Queue Element(queue=w1172, timeout in ms (-1)=0, error in (no error)=w1171) -> (queue out=w1170:refnum<queue>, element=w1175:T7, error out=w1169:errorcluster)  [unwired: 1 out]
        n409 = Not Equal?(x=T7 "Busy" ("Cmd"), y=w1175) -> (x != y?=w1173:bool)
        n410 = case shown="True" w1173 {
          tunnel: w1170 -> [w1177 w1185]
          tunnel: w1169 -> [w1176 w1186]
          tunnel: [w1177 w1184] -> w1168
          tunnel: [w1176 w1187] -> w1167
          tunnel: w1164 -> [_ w1188]
          frame False {
          }
          frame True {
            n411 = case shown="True" w1188 {
              tunnel: [w1192 w1203] -> w1187
              tunnel: w1186 -> [w1199 w1230]
              tunnel: w1185 -> [w1200 w1231]
              tunnel: [w1191 w1202] -> w1184
              frame False {
                n412 = Enqueue Element(queue=w1200, element=T7 "p" ("Cmd"), error in (no error)=w1199) -> (queue out=w1196:refnum<queue>, error out=w1195:errorcluster)  [unwired: 1 in, 1 out]
                n413 = Enqueue Element(queue=w1196, element=T7 "G" ("Cmd"), error in (no error)=w1195) -> (queue out=w1194:refnum<queue>, error out=w1193:errorcluster)  [unwired: 1 in, 1 out]
                n414 = Enqueue Element(queue=w1194, element=T7 "g" ("Cmd"), error in (no error)=w1193) -> (queue out=w1191:refnum<queue>, error out=w1192:errorcluster)  [unwired: 1 in, 1 out]
              }
              frame True {
                n415 = Enqueue Element(queue=w1231, element=T7 "P" ("Cmd"), error in (no error)=w1230) -> (queue out=w1224:refnum<queue>, error out=w1223:errorcluster)  [unwired: 1 in, 1 out]
                n416 = Enqueue Element(queue=w1224, element=T7 "F" ("Cmd"), error in (no error)=w1223) -> (queue out=w1228:refnum<queue>, error out=w1229:errorcluster)  [unwired: 1 in, 1 out]
                n417 = Enqueue Element(queue=w1228, element=T7 "A" ("Cmd"), error in (no error)=w1229) -> (queue out=w1209:refnum<queue>, error out=w1208:errorcluster)  [unwired: 1 in, 1 out]
                n418 = Enqueue Element(queue=w1209, element=T7 "T" ("Cmd"), error in (no error)=w1208) -> (queue out=w1211:refnum<queue>, error out=w1210:errorcluster)  [unwired: 1 in, 1 out]
                n419 = Enqueue Element(queue=w1211, element=T7 "t" ("Cmd"), error in (no error)=w1210) -> (queue out=w1206:refnum<queue>, error out=w1207:errorcluster)  [unwired: 1 in, 1 out]
                n420 = Enqueue Element(queue=w1206, element=T7 "M" ("Cmd"), error in (no error)=w1207) -> (queue out=w1220:refnum<queue>, error out=w1219:errorcluster)  [unwired: 1 in, 1 out]
                n421 = Enqueue Element(queue=w1220, element=T7 "G" ("Cmd"), error in (no error)=w1219) -> (queue out=w1221:refnum<queue>, error out=w1222:errorcluster)  [unwired: 1 in, 1 out]
                n422 = Enqueue Element(queue=w1221, element=T7 "g" ("Cmd"), error in (no error)=w1222) -> (queue out=w1216:refnum<queue>, error out=w1215:errorcluster)  [unwired: 1 in, 1 out]
                n423 = Enqueue Element(queue=w1216, element=T7 "EEPROM_Pconsts" ("Cmd"), error in (no error)=w1215) -> (queue out=w1205:refnum<queue>, error out=w1204:errorcluster)  [unwired: 1 in, 1 out]
                n424 = Enqueue Element(queue=w1205, element=T7 "C" ("Cmd"), error in (no error)=w1204) -> (queue out=w1202:refnum<queue>, error out=w1203:errorcluster)  [unwired: 1 in, 1 out]
              }
            }
            n425 = local write "ACK 1"(FALSE ("ACK 1")) -> ()
            n426 = local write "ACK 5"(FALSE ("ACK 8")) -> ()
            n427 = local write "ACK 2"(FALSE ("ACK 6")) -> ()
            n428 = local write "ACK 6"(FALSE ("ACK 6")) -> ()
            n429 = local write "ACK 3"(FALSE ("ACK 8")) -> ()
            n430 = local write "ACK 7"(FALSE ("ACK 6")) -> ()
            n431 = local write "ACK 4"(FALSE ("Done")) -> ()
          }
        }
      }
      event "Stop UI": Value Change {
        # "only queue msg if not busy"
        n432 = event-data() -> ()  [unwired: 1 in, 2 out]
        n433 = Preview Queue Element(queue=w1237, timeout in ms (-1)=0, error in (no error)=w1238) -> (queue out=w1236:refnum<queue>, element=w1241:T7, error out=w1235:errorcluster)  [unwired: 1 out]
        n434 = Not Equal?(x=T7 "Busy" ("Cmd"), y=w1241) -> (x != y?=w1234:bool)
        n435 = case shown="True" w1234 {
          tunnel: [w1246 w1260] -> w1243
          tunnel: [w1245 w1259] -> w1242
          tunnel: w1236 -> [w1246 w1257]
          tunnel: w1235 -> [w1245 w1256]
          tunnel: [TRUE FALSE] -> w1233
          frame False {
          }
          frame True {
            n436 = local write "ACK 1"(FALSE ("ACK 1")) -> ()
            n437 = local write "ACK 5"(FALSE ("ACK 8")) -> ()
            n438 = local write "ACK 2"(FALSE ("ACK 6")) -> ()
            n439 = local write "ACK 6"(FALSE ("ACK 6")) -> ()
            n440 = local write "ACK 3"(FALSE ("ACK 8")) -> ()
            n441 = local write "ACK 7"(FALSE ("ACK 6")) -> ()
            n442 = Enqueue Element(queue=w1257, element=T7 "Exit" ("Cmd"), error in (no error)=w1256) -> (queue out=w1260:refnum<queue>, error out=w1259:errorcluster)  [unwired: 1 in, 1 out]
            n443 = local write "ACK 4"(FALSE ("Done")) -> ()
            n444 = local write "ACK 8"(FALSE ("Done")) -> ()
          }
        }
      }
      event "Reset": Value Change {
        # "only queue msg if not busy"
        n445 = event-data() -> ()  [unwired: 1 in, 2 out]
        n446 = Preview Queue Element(queue=w1265, timeout in ms (-1)=0, error in (no error)=w1264) -> (queue out=w1268:refnum<queue>, element=w1271:T7, error out=w1267:errorcluster)  [unwired: 1 out]
        n447 = Not Equal?(x=T7 "Busy" ("Cmd"), y=w1271) -> (x != y?=w1269:bool)
        n448 = case shown="True" w1269 {
          tunnel: w1268 -> [w1273 w1311]
          tunnel: w1267 -> [w1272 w1310]
          tunnel: [w1273 w1281] -> w1262
          tunnel: [w1272 w1282] -> w1263
          frame False {
          }
          frame True {
            n449 = Enqueue Element(queue=w1311, element=T7 "R" ("Cmd"), error in (no error)=w1310) -> (queue out=w1299:refnum<queue>, error out=w1298:errorcluster)  [unwired: 1 in, 1 out]
            n450 = local write "ACK 1"(FALSE ("ACK 1")) -> ()
            n451 = local write "ACK 5"(FALSE ("ACK 8")) -> ()
            n452 = Enqueue Element(queue=w1299, element=T7 "F" ("Cmd"), error in (no error)=w1298) -> (queue out=w1307:refnum<queue>, error out=w1297:errorcluster)  [unwired: 1 in, 1 out]
            n453 = local write "ACK 2"(FALSE ("ACK 6")) -> ()
            n454 = local write "ACK 6"(FALSE ("ACK 6")) -> ()
            n455 = Enqueue Element(queue=w1307, element=T7 "A" ("Cmd"), error in (no error)=w1297) -> (queue out=w1289:refnum<queue>, error out=w1288:errorcluster)  [unwired: 1 in, 1 out]
            n456 = Enqueue Element(queue=w1289, element=T7 "T" ("Cmd"), error in (no error)=w1288) -> (queue out=w1291:refnum<queue>, error out=w1290:errorcluster)  [unwired: 1 in, 1 out]
            n457 = local write "ACK 3"(FALSE ("ACK 8")) -> ()
            n458 = local write "ACK 7"(FALSE ("ACK 6")) -> ()
            n459 = Enqueue Element(queue=w1291, element=T7 "t" ("Cmd"), error in (no error)=w1290) -> (queue out=w1287:refnum<queue>, error out=w1286:errorcluster)  [unwired: 1 in, 1 out]
            n460 = local write "ACK 4"(FALSE ("Done")) -> ()
            n461 = Enqueue Element(queue=w1287, element=T7 "M" ("Cmd"), error in (no error)=w1286) -> (queue out=w1303:refnum<queue>, error out=w1296:errorcluster)  [unwired: 1 in, 1 out]
            n462 = Enqueue Element(queue=w1303, element=T7 "G" ("Cmd"), error in (no error)=w1296) -> (queue out=w1304:refnum<queue>, error out=w1295:errorcluster)  [unwired: 1 in, 1 out]
            n463 = Enqueue Element(queue=w1304, element=T7 "g" ("Cmd"), error in (no error)=w1295) -> (queue out=w1300:refnum<queue>, error out=w1294:errorcluster)  [unwired: 1 in, 1 out]
            n464 = Enqueue Element(queue=w1300, element=T7 "EEPROM_Pconsts" ("Cmd"), error in (no error)=w1294) -> (queue out=w1284:refnum<queue>, error out=w1283:errorcluster)  [unwired: 1 in, 1 out]
            n465 = Enqueue Element(queue=w1284, element=T7 "C" ("Cmd"), error in (no error)=w1283) -> (queue out=w1281:refnum<queue>, error out=w1282:errorcluster)  [unwired: 1 in, 1 out]
          }
        }
      }
      event "Start streaming": Value Change {
        # "only queue msg if not busy AND main power is on"
        n466 = event-data() -> ()  [unwired: 1 in, 2 out]
        n467 = local read "System status"() -> (w1314:T5)
        n468 = Unbundle By Name(w1314) -> ("Main power"=w1313:bool)
        n469 = Preview Queue Element(queue=w1320, timeout in ms (-1)=0, error in (no error)=w1317) -> (queue out=w1323:refnum<queue>, element=w1326:T7, error out=w1322:errorcluster)  [unwired: 1 out]
        n470 = Not Equal?(x=T7 "Busy" ("Cmd"), y=w1326) -> (x != y?=w1324:bool)
        n471 = And(x=w1313, y=w1324) -> (x .and. y?=w1315:bool)
        n472 = case shown="True" w1315 {
          tunnel: w1323 -> [w1328 w1332]
          tunnel: w1322 -> [w1327 w1331]
          tunnel: [w1328 w1329] -> w1319
          tunnel: [w1327 w1330] -> w1318
          frame False {
          }
          frame True {
            n473 = Enqueue Element(queue=w1332, element=T7 "S" ("Cmd"), error in (no error)=w1331) -> (queue out=w1329:refnum<queue>, error out=w1330:errorcluster)  [unwired: 1 in, 1 out]
          }
        }
      }
      event "Apply settings 1": Value Change {
        # "only queue msg if not busy"
        n474 = event-data() -> ()  [unwired: 1 in, 2 out]
        n475 = Preview Queue Element(queue=w1338, timeout in ms (-1)=0, error in (no error)=w1337) -> (queue out=w1341:refnum<queue>, element=w1344:T7, error out=w1340:errorcluster)  [unwired: 1 out]
        n476 = Not Equal?(x=T7 "Busy" ("Cmd"), y=w1344) -> (x != y?=w1342:bool)
        n477 = case shown="True" w1342 {
          tunnel: w1341 -> [w1346 w1360]
          tunnel: w1340 -> [w1345 w1359]
          tunnel: [w1346 w1349] -> w1334
          tunnel: [w1345 w1348] -> w1335
          frame False {
          }
          frame True {
            n478 = local write "ACK 2"(FALSE ("ACK 1")) -> ()
            n479 = Enqueue Element(queue=w1360, element=T7 "T" ("Cmd"), error in (no error)=w1359) -> (queue out=w1357:refnum<queue>, error out=w1356:errorcluster)  [unwired: 1 in, 1 out]
            n480 = Enqueue Element(queue=w1357, element=T7 "t" ("Cmd"), error in (no error)=w1356) -> (queue out=w1354:refnum<queue>, error out=w1355:errorcluster)  [unwired: 1 in, 1 out]
            n481 = Enqueue Element(queue=w1354, element=T7 "M" ("Cmd"), error in (no error)=w1355) -> (queue out=w1351:refnum<queue>, error out=w1350:errorcluster)  [unwired: 1 in, 1 out]
            n482 = Enqueue Element(queue=w1351, element=T7 "g" ("Cmd"), error in (no error)=w1350) -> (queue out=w1349:refnum<queue>, error out=w1348:errorcluster)  [unwired: 1 in, 1 out]
          }
        }
      }
      event "Apply settings 2": Value Change {
        # "only queue msg if not busy"
        n483 = event-data() -> ()  [unwired: 1 in, 2 out]
        n484 = Preview Queue Element(queue=w1366, timeout in ms (-1)=0, error in (no error)=w1365) -> (queue out=w1369:refnum<queue>, element=w1372:T7, error out=w1368:errorcluster)  [unwired: 1 out]
        n485 = Not Equal?(x=T7 "Busy" ("Cmd"), y=w1372) -> (x != y?=w1370:bool)
        n486 = case shown="True" w1370 {
          tunnel: w1369 -> [w1374 w1394]
          tunnel: w1368 -> [w1373 w1393]
          tunnel: [w1374 w1375] -> w1363
          tunnel: [w1373 w1376] -> w1364
          frame False {
          }
          frame True {
            n487 = local write "ACK 3"(FALSE ("ACK 1")) -> ()
            n488 = Enqueue Element(queue=w1394, element=T7 "O" ("Cmd"), error in (no error)=w1393) -> (queue out=w1390:refnum<queue>, error out=w1389:errorcluster)  [unwired: 1 in, 1 out]
            n489 = Enqueue Element(queue=w1390, element=T7 "G" ("Cmd"), error in (no error)=w1389) -> (queue out=w1378:refnum<queue>, error out=w1377:errorcluster)  [unwired: 1 in, 1 out]
            n490 = Enqueue Element(queue=w1378, element=T7 "F" ("Cmd"), error in (no error)=w1377) -> (queue out=w1382:refnum<queue>, error out=w1383:errorcluster)  [unwired: 1 in, 1 out]
            n491 = Enqueue Element(queue=w1382, element=T7 "A" ("Cmd"), error in (no error)=w1383) -> (queue out=w1380:refnum<queue>, error out=w1379:errorcluster)  [unwired: 1 in, 1 out]
            n492 = Enqueue Element(queue=w1380, element=T7 "M" ("Cmd"), error in (no error)=w1379) -> (queue out=w1387:refnum<queue>, error out=w1388:errorcluster)  [unwired: 1 in, 1 out]
            n493 = Enqueue Element(queue=w1387, element=T7 "EEPROM_Pconsts" ("Cmd"), error in (no error)=w1388) -> (queue out=w1375:refnum<queue>, error out=w1376:errorcluster)  [unwired: 1 in, 1 out]
          }
        }
      }
      event "Refresh sys. status": Value Change {
        # "only queue msg if not busy"
        n494 = event-data() -> ()  [unwired: 1 in, 2 out]
        n495 = Preview Queue Element(queue=w1400, timeout in ms (-1)=0, error in (no error)=w1399) -> (queue out=w1403:refnum<queue>, element=w1406:T7, error out=w1402:errorcluster)  [unwired: 1 out]
        n496 = Not Equal?(x=T7 "Busy" ("Cmd"), y=w1406) -> (x != y?=w1404:bool)
        n497 = case shown="True" w1404 {
          tunnel: w1403 -> [w1408 w1416]
          tunnel: w1402 -> [w1407 w1415]
          tunnel: [w1408 w1413] -> w1398
          tunnel: [w1407 w1412] -> w1397
          frame False {
          }
          frame True {
            n498 = local write "ACK 5"(FALSE ("ACK 1")) -> ()
            n499 = Enqueue Element(queue=w1416, element=T7 "G" ("Cmd"), error in (no error)=w1415) -> (queue out=w1414:refnum<queue>, error out=w1411:errorcluster)  [unwired: 1 in, 1 out]
            n500 = Enqueue Element(queue=w1414, element=T7 "g" ("Cmd"), error in (no error)=w1411) -> (queue out=w1413:refnum<queue>, error out=w1412:errorcluster)  [unwired: 1 in, 1 out]
          }
        }
      }
      event "Apply settings 3": Value Change {
        # "only queue msg if not busy"
        n501 = event-data() -> ()  [unwired: 1 in, 2 out]
        n502 = Preview Queue Element(queue=w1422, timeout in ms (-1)=0, error in (no error)=w1421) -> (queue out=w1425:refnum<queue>, element=w1428:T7, error out=w1424:errorcluster)  [unwired: 1 out]
        n503 = Not Equal?(x=T7 "Busy" ("Cmd"), y=w1428) -> (x != y?=w1426:bool)
        n504 = case shown="True" w1426 {
          tunnel: w1425 -> [w1430 w1435]
          tunnel: w1424 -> [w1429 w1434]
          tunnel: [w1430 w1432] -> w1419
          tunnel: [w1429 w1433] -> w1420
          frame False {
          }
          frame True {
            n505 = local write "ACK 4"(FALSE ("ACK 1")) -> ()
            n506 = Enqueue Element(queue=w1435, element=T7 "C" ("Cmd"), error in (no error)=w1434) -> (queue out=w1432:refnum<queue>, error out=w1433:errorcluster)  [unwired: 1 in, 1 out]
          }
        }
      }
      event "Write ASCII datalog": Value Change {
        # "only queue msg if not busy"
        n507 = event-data() -> ()  [unwired: 1 in, 2 out]
        n508 = Preview Queue Element(queue=w1441, timeout in ms (-1)=0, error in (no error)=w1440) -> (queue out=w1444:refnum<queue>, element=w1447:T7, error out=w1443:errorcluster)  [unwired: 1 out]
        n509 = Not Equal?(x=T7 "Busy" ("Cmd"), y=w1447) -> (x != y?=w1445:bool)
        n510 = case shown="True" w1445 {
          tunnel: w1444 -> [w1449 w1453]
          tunnel: w1443 -> [w1448 w1452]
          tunnel: [w1449 w1450] -> w1439
          tunnel: [w1448 w1451] -> w1438
          frame False {
          }
          frame True {
            n511 = local write "ASCII done"(FALSE ("ACK 1")) -> ()
            n512 = Enqueue Element(queue=w1453, element=T7 "convert_datalogs" ("Cmd"), error in (no error)=w1452) -> (queue out=w1450:refnum<queue>, error out=w1451:errorcluster)  [unwired: 1 in, 1 out]
          }
        }
      }
    }
  }
  n513 = Merge Errors(w32, w30) -> (w33:errorcluster)
  n514 = Release Queue(queue=w31, error in (no error)=w33) -> (error out=w17:errorcluster)  [unwired: 1 in, 2 out]
  n515 = Merge Errors(w17, w18) -> (w19:errorcluster)
  n516 = local write "Error"(w19) -> ()
